vi "Dashboard Main.vi"() -> ()   [LabVIEW 2013]
uses:
  Common Code/Shooter State.ctl
  Common Code/Dashboard UDP/Camera Controls.ctl
  Common Code/Dashboard UDP/Gyro Controls.ctl
  Common Code/Dashboard UDP/PID Params.ctl
  Common Code/Dashboard UDP/Auton Controls.ctl
  Common Code/Dashboard UDP/Shooter Controls.ctl
  Common Code/Dashboard UDP/Encoder Controls.ctl
  Common Code/Dashboard UDP/Auto Shift Controls.ctl
  Common Code/Dashboard UDP/Roller Controls.ctl
  Common Code/Dashboard UDP/Shooter Indicators.ctl
  Common Code/Dashboard UDP/Auton Indicators.ctl
  Common Code/Dashboard UDP/Roller Indicators.ctl
  Common Code/IR Logic State.ctl
  Common Code/Dashboard UDP/Drive Indicators.ctl
  Common Code/Dashboard UDP/Halo Indicators.ctl
  Robot Code/Sensors/Encoder Data.ctl
  Robot Code/Sensors/Single Encoder Data.ctl
  Common Code/Vision Mode.ctl
  Common Code/Dashboard UDP/Fieldcentric Controls.ctl
  Common Code/Dashboard UDP/Roll Maneuver.ctl
  Robot Code/Drivetrain/DT Mode.ctl
  Common Code/Dashboard UDP Packet.ctl
  Common Code/Dashboard UDP/Omni Packet.ctl
  Common Code/Dashboard UDP/Indicator Packet.ctl
  <vilib>/event_ctls.llb/eventvkey.ctl
  Common Code/Change Detect Int.vi
  Common Code/Change Detect Double.vi
  Robot Code/Utilities/TimeManager.vi
  Common Code/Change Detect Boolean.vi
  <vilib>/Rock Robotics/WPI/Dashboard/WPI_DashboardLogging Global.vi
  <vilib>/Utility/config.llb/Write Key (String).vi
  <vilib>/Utility/config.llb/Write Key (I32).vi
  <vilib>/Utility/config.llb/NI_LVConfig.lvlib
panel:
  out "Maneuver Gyro Data":dbl[](array[numeric])
  in  "Shooter High":bool
  in  "PSI Good":bool
  in  "Shooter Ready":bool
  in  "Shooter State":T1
  in  "Color Components old":T2={"Hue"={70.0, 125.0}, "Sat"={39.0, 255.0}, "Val"={115.0, 255.0}} {"Val" scale=0.0..255.0; "Sat" scale=0.0..255.0; "Hue" scale=0.0..255.0 scale format="%#_3g"}
  out "Prefs Status":string
  out "High Priority User Data":string
  in  "Pressure/Blink Time":dbl=-1.0 caption="Blink (ms)"
  in  "Pressure/Deflicker":dbl=-1.0 caption="Deflicker (ms)"
  in  "Pressure/PID Setpoints D":dbl=-1.0 caption="D"
  in  "Pressure/PID Setpoints I":dbl=-1.0 caption="I"
  in  "Pressure/PID Setpoints P":dbl=-1.0 caption="P"
  in  "Pressure/PID Setpoints min":dbl=-1.0 caption="min"
  in  "Pressure/PID Setpoints max":dbl=-1.0 caption="max"
  in  "Pressure/Blink PSI Threshold":dbl=-1.0 caption="Blink Threshold"
  in  "Pressure/PSI Tolerance":dbl=-1.0 caption="Shoot\nThreshold"
  in  "Reload":bool
  in  "Save":bool
  out "Camera 2 IP":string="10.6.24.12"
  out "Camera IP":string="10.6.24.11"
  out "Heartbeat":dbl
  out "Connection LED":bool
  in  "stop":bool
  in  "Save Constants File":bool caption="Save"
  in  "Reload Constants File":bool caption="Reload"
  out "Image Message":string="Timeout in Camera Communications"
  in  "Rec Mode":enum32{"Stop", "Record", "Playback"}(radio)
  in  "Dashboard Tab":T3(tab)
  out "Shooter Retracted":bool caption="Retracted"
  out "Halo Mode":bool
  out "Roller Mode":bool
  out "Halo Indicators 2":T4
  out "Shooter State Indicator":bool
  out "Pressure/Shooter":dbl caption="Shooter"
  out "Shooter/High":bool caption="Pressure Setting"
  out "Pressure/Line":dbl(slide)=-1.0 caption="Tank" scale=50.0..120.0
  out "Pressure/Shooter":dbl(knob)=-1.0 caption="Shooter PSI" scale=30.0..60.0
  out "Shooter/State":T1
  out "Shooter/Trigger":bool caption="Trigger"
  out "Shooter/Release":bool caption="Release"
  out "Shooter/Add":bool caption="Add"
  out "Shooter/Ready":bool caption="Ready"
  out "Gyro Heading":dbl(knob) caption="Gyro" scale=0.0..359.0
  out "Roller Indicators 2":T5 caption="Rollers"
  out "Drive Indicators 2":T7 caption="Drive" {"Roller/Back Output" scale=-1.0..1.0; "Roller/Front Output" scale=-1.0..1.0; "Drive/Translation X" scale=-1.0..1.0; "Drive/Steer" scale=-1.0..1.0; "Drive/Throttle" scale=-1.0..1.0}
  out "Gyro Heading":dbl(knob) caption="Gyro" scale=0.0..359.0
  in  "Disable Compressor":bool caption="Disable\nCompressor"
  in  "IR Halo Sustain Time":dbl caption="IR Halo Sustain"
  out "Halo Indicators":T8
  in  "Encoder":T9={"Encoders/Reset"=FALSE, "Encoders/Omni Constant"=0.000546, "Encoders/Omni Tick Constant"=10.27628431, "Encoders/Left Constant"=0.000546, "Encoders/Right Constant"=0.000546, "Encoders/Right Tick Constant"=1.0}
  out "Drive/Gear":dbl caption="Gear"
  in  "Pressure/Compressor Delay":dbl=500.0 caption="Delay"
  in  "Pressure/Compressor Min Voltage":dbl=7.0 caption="Min Volts"
  in  "Drive/Ramp X":dbl=250.0 caption="Ramp X (ms)"
  in  "Drive/Ramp Y":dbl=250.0 caption="Ramp Y (ms)"
  out "IR Dist/Line Detected Right":bool caption="Right Line"
  out "IR Dist/Line Detected Left":bool caption="Left Line"
  in  "Drive/Battery Cutoff":dbl=6.0 caption="Drive Min Volts"
  in  "Shooter":T10={"Shooter/Reset Time"=500.0, "Shooter/Release Delay"=150.0, "Shooter/Pressure Steady Time"=0.0, "Shooter/Misfire Delay"=2000.0, "Shooter/Ball Settle Time"=500.0, "Shooter/Line IR Delay"=300.0, "Pressure/Upper PSI Time"=500.0, "Pressure/Lower PSI Time"=500.0, "Shooter/Punch Delay"=-150.0, "Shooter/Target Pressure"=43.0, "Pressure/Line B"=-57.077, "Pressure/Line M"=33.41, "Pressure/Shooter M"=33.41, "Pressure/Shooter B"=-57.077, "Halo Time"=150.0, "Soft Release Delay"=0.0, "Soft Unpin Delay"=0.0, "Soft Shoot Delay"=0.0, "Toss Release Time"=0.0} caption="Soft Shoot"
  in  "Auto Shift":T11={"AutoShift/Upshift Throttle Accel"=-2.0, "AutoShift/Speed Threshold"=5.0, "AutoShift/Upshift Throttle"=0.8, "AutoShift/Upshift Accel"=0.5, "AutoShift/Downshift Accel"=-1.2, "AutoShift/Downshift Throttle"=0.15, "AutoShift/Delay"=1000.0, "AutoShift/Enabled"=TRUE}
  in  "Rollers":T12={"Roller/Load IRs Verify Time"=150.0, "Roller/Center IR Latch Time"=500.0, "Roller/Speed Front"=0.8, "Roller/Speed Back"=0.3, "Roller/Entry Timeout"=750.0, "Roller/To Center Timeout"=2000.0, "Roller/Sustain Time"=5000.0, "Roller/Verify Center Time"=750.0}
  out "Shooter Indicators":T13={"Pressure/Line"=-1.0, "Pressure/Shooter"=-1.0, "Shooter/Release"=FALSE, "Shooter/Trigger"=FALSE, "Shooter/Retracted"=FALSE, "Shooter/Ready"=FALSE, "Shooter/Add"=FALSE, "Shooter/State"=enum."Wait", "Shooter/Punch"=FALSE, "Shooter/High"=FALSE, "Shooter/AutoPunch"=FALSE}
  out "Roller Indicators":T5
  out "Drive Indicators":T7 {"Roller/Back Output" scale=-1.0..1.0; "Roller/Front Output" scale=-1.0..1.0; "Drive/Translation X" scale=-1.0..1.0; "Drive/Steer" scale=-1.0..1.0; "Drive/Throttle" scale=-1.0..1.0}
  out "Encoder Data":T14 {"Omni"."Ticks" format="%#.6g"; "Right"."Ticks" format="%#.6g"; "Left"."Ticks" format="%#.6g"}
  in  "Low PSI":dbl=52.0
  in  "Center Omni Drive Delay":dbl
  in  "Controller/Strafe Correction":bool=TRUE caption="Strafe Correct"
  in  "Auton":T16={"Auton/Left Shoot X-Coord"=-4.0, "Auton/Right Shoot X-Coord"=4.0, "DistDrive/Distance Stop Threshold"=0.25, "DistDrive/Max Stop Speed"=0.5, "Auton/Back Piston Time"=500.0, "Auton/Manual Hot"=FALSE, "Auton/Manual Hot Right"=FALSE, "Default X PID"={"max"=1.0, "min"=-1.0, "P"=0.36, "I"=0.0, "D"=0.0}, "Default Y PID"={"max"=1.0, "min"=-1.0, "P"=0.7, "I"=0.0, "D"=0.001}, "Half Over Delay"=0.0}
  out "Auton/Files":string
  out "Auton Indicators":T18
  out "Vision Mode":T19 caption="Vision Mode (Reported by Robot)"
  in  "Normal Vision":bool=TRUE
  in  "Extreme Left":bool
  in  "Extreme Right":bool
  out "Vision Mode Cam":T19 caption="Reported Vision Mode"
  in  "Camera":T20={"Camera/View Angle X"=66.5, "Camera/Goal Track Timeout"=120.0, "Camera/View Angle Y"=49.0, "Camera/Goal Exposure"=0.0, "Camera/Vision Receive Timeout"=120.0, "Camera/Offset 1"=-35.0, "Camera/Offset 2"=35.0}
  in  "Cam 2 Enable":bool=TRUE
  out "Auton/Right Hot":bool
  out "Auton/Left Hot":bool
  out "Cam2 FPS":dbl format="%#.1g"
  out "Cam2 Mbps":dbl format="%#.1g"
  out "Cam2 LED":bool
  in  "Camera Settings":T21={"Frame Rate"=30, "Compression"=30, "Size"=1} {"Frame Rate" scale=1.0..30.0; "Size" items=["640x480", "320x240", "160x120"]}
  out "Camera Image":T22(plugin-control)
  in  "Cam 1 Enable":bool=TRUE
  out "Camera Image 2":T22(plugin-control)
  out "Mbps 2":bool
  out "Cam1 Mbps":dbl format="%#.1g"
  out "Cam1 FPS":dbl format="%#.1g"
  in  "DB Camera Config":bool
  in  "Test Slider":dbl(slide) scale=0.0..100.0 scale format="%#_3g"
  in  "On/Off":bool caption="Solenoid"
  in  "Test Name":u16(ring) items=["Select the test to run...", "Example Test", "-------------------------------", "List of tests is built in robot code.", "Replace with your own automated tests."]
  in  "Test Tree":string(tree)
  in  "Motor":cluster{"Value":dbl, "Enable":bool} {"Value" scale=-1.0..1.0 scale format="%#_3g"}
  out "Progress":T23 {"Test Progress" scale=0.0..100.0}
  in  "Rev/Fwd":cluster{"Forward":bool, "Reverse":bool}
  in  "Test Ring":u16(ring) items=["Auto", "Fixed indoor", "Fixed outdoor 1", "Fixed outdoor 2", "Fixed fluorescent 1", "Fixed fluorescent 2", "Hold current"]
  out "Tree":string(tree)
  in  "Listbox":i32(listbox)
  out "Warnings List":string
  out "Preferences Count":i32
  in  "Gyro":T24={"Gyro/Angle Tolerance"=2.0, "Gyro/Steer Closeness Threshold"=10.0, "Steer PID"={"max"=0.8, "min"=-0.8, "P"=0.04, "I"=0.0, "D"=0.0}, "Steer Close PID"={"max"=0.7, "min"=-0.7, "P"=0.04, "I"=0.0, "D"=0.002}}
  out "Gyro/In Range":bool
  out "Gyro/Steer Target":dbl
  out "Gyro Heading":dbl(knob) scale=0.0..359.0
  out "Vision Mode Goal Tab":T19 caption="Vision Mode"
  in  "Cam 1/2":bool
  out "Goal Mask":T22(plugin-control)
  out "Goal Camera Image":T22(plugin-control)
  in  "Score Cutoff":dbl(slide)=54.248366013071895 scale=0.0..100.0
  in  "HSV Filter":T25={"Hue min"=100.0, "Hue max"=125.0, "Sat min"=60.0, "Sat max"=255.0, "Lum min"=155.0, "Lum max"=255.0}
  in  "Stick Deadband":dbl
  out "Angle Graph":T26(graph)
  out "Drive Graph":cluster{i32, "Timestep(ms)":i32, dbl[][]}(graph)
  in  "Roll":T27
  in  "Fieldcentric":T28
  in  "Radius Throttle":bool
  out "Drivetrain Mode":T29
  out "Time/100ms loop exec time":dbl
  in  "Finish":bool caption="Self Destruct"
  in  "Abort":bool caption="Self Destruct"
  out "Mode":T30(ring)=enum."Auto Disabled"
  # "Pressure PID"
  # "psi"
  # "psi"
  # "Shooter"
  # "IR"
  # "Encoders"
  # "Auto Shift"
  # "Compressor"
  # "Feet"
  # "Line"
  # "Shooter"
  # "Down"
  # "Up"
  # "IR"
  # "Left"
  # "Front"
  # "Right"
  # "Battery"
  # "2"
  # "1"
  # "Goal Tracking"
  # "DRIVER [USB 1]"
  # "Manipulator [USB 2]"
  # "DRIVER [USB 1]"
  # "Manipulator [USB 2]"
  # "JOYSTICK"
  # "CONTROLS"
  # "GAMEPAD"
  # "CONTROLS"
  # "GAMEPAD"
  # "CONTROLS"
  # "GAMEPAD"
  # "CONTROLS"
  # "Joystick"
  # "A 1-X    \tThrottle\t\nA 2-Y     Lateral Throttle (Omni)\nA 3-Z     Spin\nA +/-     Omni Traction Switch\n\n1\t            Gear Shift (INA)\n2\t            Shoot (RAS)\n3\t            Collect Ball (Front)\t(INA)\n4\t            Collect Ball (Rear) (INA)\n5\t            Trigger\n6\t            Reset Gyro\n7\t            Front Arm Up/Down \n8\t            Back Arm Up/Down\n9\t            F Roller In\n10\t\t         R Roller In\n11           F Roller Out\n12           R Roller Out\n\t\t\nUP\t           Add Pressure\t\nDOWN\t    Release Pressure\t\nLEFT\t        Goal Offset LEFT\nRIGHT\t\t    Goal Offset RIGHT"
  # "11           \t\n12\t\t\n\n\n\n1\t\t\n2\t            \n3\t            Warmup\t\n4\t\t\n5             \n6\t            \t\n7\t            \n8\t\n9\t            Camera Search\t*\n10\t          Auto Ball\t*\n11\t          \t\n12\t\n\t\nUP\t\t\nDOWN\t\t\nLEFT\t\t\nRIGHT"
  # "Joystick"
  # "11    \t      Throttle\t\n12\t          Steer\n\n1\t            Roll maneuver left\n2\t            Shoot\t& (AS)\n3\t            \tRoll maneuver right\n4\t            Goal Steer\t& (AS)\n5\t            Manual low gear / Gear          \n               shift\n6\t            Omni Toggle\t\n7\t            Strafe Left \n8\t            Strafe Right\n9\t             \n10\t\t\n11          \t\n12\n\t\n\n\t\nUP\t          \t\nDOWN\t    \t\nLEFT\t        \t\nRIGHT"
  # "11        Y-High/Low PSI Set\n12\t  R= Hold Ball L=Carry Two               \n1\t\t        SHIFT Alt Ctrl [...]\n2\t         Shoot\t\n3\t         Ready Shooter\t\n4\t\t        Invert Halo\n5          Front Roller-Fwds\n                [manual Trigger*]\n6\t    \t\n7\t         Front Roller-Backwds\t\n                [Line Shoot]\n8\t     \n9\t        Auto Halo* \n         [Manual Halo Setting] \n10\t       Auto Roller\t*\n11\t      \t\n12\t       Recal Gyro (only when    disabled)\n\nUP\t\t       Load Front [+ Air]\nDOWN\t Reset Load [- Air]\nLEFT\t\t    Load Front [Reset Air]\nRIGHT   Toss Ball"
  # "Buttons"
  # "Buttons"
  # "D-Pad"
  # "D-Pad"
  # "(INA) If Not Automated"
  # "* Toggle"
  # "AUTON SELECT: With robot disabled, press button 9 + button 2 to go down file list\n                                                                         button 9 + button 4 to go up file list"
  # "(RAS) Runs Automatic Sequence"
  # "* Toggle"
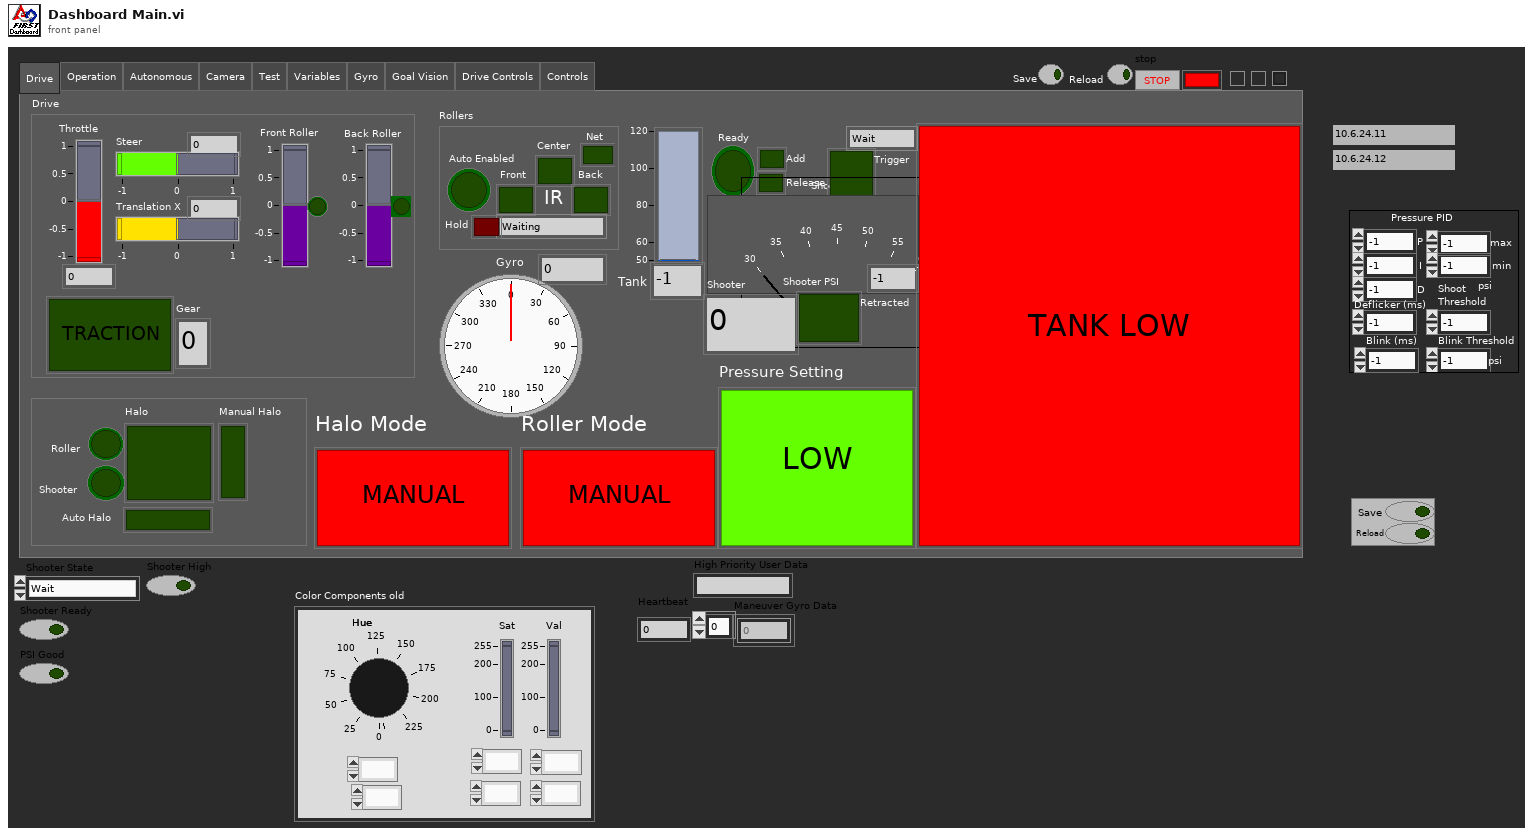
[diagram p1: front panel]
types:
  T1 = typedef "Shooter State.ctl" = enum16{"Wait", "Fill Piston", "Lift Halo", "Trigger", "Reset", "Soft Release", "Soft Unpin", "Soft Refill", "Soft Shoot", "Toss Prep", "Toss Release"}
  T2 = cluster{"Hue":cluster{dbl, dbl}, "Sat":cluster{dbl, dbl}, "Val":cluster{dbl, dbl}}
  T3 = enum32{"Drive", "Operation", "Autonomous", "Camera", "Test", "Variables", "Gyro", "Goal Vision", "Drive Controls", "Controls"}
  T4 = cluster{"Halo":bool, "Roller Halo":bool, "Shooter Halo":bool, "Auto Halo":bool, "Manual Halo":bool}
  T5 = typedef "Roller Indicators.ctl" = cluster{"Roller/Front IR":bool, "Roller/Center IR":bool, "Roller/Back IR":bool, "Roller/IR State":T6, "Roller/Auto Enabled":bool, "Roller/Hold":bool, "Roller/Net Solenoid":bool}
  T6 = typedef "IR Logic State.ctl" = enum16{"Waiting", "Requested", "Loading", "Full", "Wait for Center", "Carry", "Full Carry", "Holding"}
  T7 = typedef "Drive Indicators.ctl" = cluster{"Drive/Throttle":dbl, "Drive/Steer":dbl, "Drive/Translation X":dbl, "Drive/Omni":bool, "Roller/Front Output":dbl, "Roller/Back Output":dbl, "Roller/Front Solenoid":bool, "Roller/Back Solenoid":bool, "Drive/Gear":dbl}
  T8 = typedef "Halo Indicators.ctl" = cluster{"Halo":bool, "Roller Halo":bool, "Shooter Halo":bool, "Auto Halo":bool, "Manual Halo":bool}
  T9 = typedef "Encoder Controls.ctl" = cluster{"Encoders/Reset":bool, "Encoders/Omni Constant":dbl, "Encoders/Omni Tick Constant":dbl, "Encoders/Left Constant":dbl, "Encoders/Right Constant":dbl, "Encoders/Right Tick Constant":dbl}
  T10 = typedef "Shooter Controls.ctl" = cluster{"Shooter/Reset Time":dbl, "Shooter/Release Delay":dbl, "Shooter/Pressure Steady Time":dbl, "Shooter/Misfire Delay":dbl, "Shooter/Ball Settle Time":dbl, "Shooter/Line IR Delay":dbl, "Pressure/Upper PSI Time":dbl, "Pressure/Lower PSI Time":dbl, "Shooter/Punch Delay":dbl, "Shooter/Target Pressure":dbl, "Pressure/Line B":dbl, "Pressure/Line M":dbl, "Pressure/Shooter M":dbl, "Pressure/Shooter B":dbl, "Halo Time":dbl, "Soft Release Delay":dbl, "Soft Unpin Delay":dbl, "Soft Shoot Delay":dbl, "Toss Release Time":dbl}
  T11 = typedef "Auto Shift Controls.ctl" = cluster{"AutoShift/Upshift Throttle Accel":dbl, "AutoShift/Speed Threshold":dbl, "AutoShift/Upshift Throttle":dbl, "AutoShift/Upshift Accel":dbl, "AutoShift/Downshift Accel":dbl, "AutoShift/Downshift Throttle":dbl, "AutoShift/Delay":dbl, "AutoShift/Enabled":bool}
  T12 = typedef "Roller Controls.ctl" = cluster{"Roller/Load IRs Verify Time":dbl, "Roller/Center IR Latch Time":dbl, "Roller/Speed Front":dbl, "Roller/Speed Back":dbl, "Roller/Entry Timeout":dbl, "Roller/To Center Timeout":dbl, "Roller/Sustain Time":dbl, "Roller/Verify Center Time":dbl}
  T13 = typedef "Shooter Indicators.ctl" = cluster{"Pressure/Line":dbl, "Pressure/Shooter":dbl, "Shooter/Release":bool, "Shooter/Trigger":bool, "Shooter/Retracted":bool, "Shooter/Ready":bool, "Shooter/Add":bool, "Shooter/State":T1, "Shooter/Punch":bool, "Shooter/High":bool, "Shooter/AutoPunch":bool}
  T14 = typedef "Encoder Data.ctl" = cluster{"Avg Distance L/R":dbl, "Avg Speed L/R":dbl, "Left":T15, "Right":T15, "Omni":T15}
  T15 = typedef "Single Encoder Data.ctl" = cluster{"Distance":dbl, "Speed":dbl, "Ticks":dbl}
  T16 = typedef "Auton Controls.ctl" = cluster{"Auton/Left Shoot X-Coord":dbl, "Auton/Right Shoot X-Coord":dbl, "DistDrive/Distance Stop Threshold":dbl, "DistDrive/Max Stop Speed":dbl, "Auton/Back Piston Time":dbl, "Auton/Manual Hot":bool, "Auton/Manual Hot Right":bool, "Default X PID":T17, "Default Y PID":T17, "Half Over Delay":dbl}
  T17 = typedef "PID Params.ctl" = cluster{"max":dbl, "min":dbl, "P":dbl, "I":dbl, "D":dbl}
  T18 = typedef "Auton Indicators.ctl" = cluster{"DistDrive/Steer":bool, "DistDrive/Y Check":bool, "Auton/Left Hot":bool, "Auton/Right Hot":bool, "DistDrive/Y Dist":dbl, "DistDrive/Y Target":dbl, "DistDrive/X Dist":dbl, "DistDrive/X Target":dbl, "Gyro Heading":dbl, "DistDrive/Steer Target":dbl, "DistDrive/X Check":bool, "Auton/Hot Found":bool, "Auton/Goals Used":dbl, "Auton/Total Commands":dbl, "Auton/Current Command":dbl, "Auton/File":dbl}
  T19 = typedef "Vision Mode.ctl" = enum16{"Normal", "Extreme Left", "Extreme Right"}
  T20 = typedef "Camera Controls.ctl" = cluster{"Camera/View Angle X":dbl, "Camera/Goal Track Timeout":dbl, "Camera/View Angle Y":dbl, "Camera/Goal Exposure":dbl, "Camera/Vision Receive Timeout":dbl, "Camera/Offset 1":dbl, "Camera/Offset 2":dbl}
  T21 = cluster{"Frame Rate":i32, "Compression":i32, "Size":u16}
  T22 = typedef "IMAQ Image.ctl" = refnum<image>
  T23 = cluster{"Test Progress":u8, "Test Progress Text":string}
  T24 = typedef "Gyro Controls.ctl" = cluster{"Gyro/Angle Tolerance":dbl, "Gyro/Steer Closeness Threshold":dbl, "Steer PID":T17, "Steer Close PID":T17}
  T25 = cluster{"Hue min":dbl, "Hue max":dbl, "Sat min":dbl, "Sat max":dbl, "Lum min":dbl, "Lum max":dbl}
  T26 = cluster{i32, "Timestep(ms)":i32, "Maneuver Gyro Data":dbl[]}[]
  T27 = typedef "Roll Maneuver.ctl" = cluster{"X 1":dbl, "Y 1":dbl, "Y 2":dbl, "X 2":dbl, "Y 3":dbl, "X 3":dbl, "Time 1":i32, "Time 2":i32, "Time 3":i32, "Angle Start":dbl, "Angle End":dbl, "Angle Linearity":dbl}
  T28 = typedef "Fieldcentric Controls.ctl" = cluster{"Relative Angle":bool, "Point Robot":bool, "X/Y ratio low":dbl, "Steering Gain":dbl, "Force Omni Down":bool, "Enable":bool, "X/Y ratio high":dbl}
  T29 = typedef "DT Mode.ctl" = enum16{"Manual", "Gyro Steer", "Distance Drive", "Fieldcentric", "Roll Maneuver", "Alt Roll Maneuver"}
  T30 = enum8{"Tele-Op Disabled", "Tele-Op Enabled", "Auto Disabled", "Auto Enabled", "Test Disabled", "Test Enabled", ""}
  T31 = typedef "Image Type" = u32
  T32 = typedef "NI_LVConfig.lvlib/Config Data RefNum.ctl" = refnum<k1>
  T33 = typedef "Goal Info.ctl" = cluster{"Found?":bool, "Target Center":cluster{"X":dbl, "Y":dbl}, "Distance (ft)":dbl, "Hot?":bool, "Left?":bool, "Camera":i16}
  T34 = cluster{"Vision Target":T33, "Vision Target":T33, "Vision Target":T33}
  T35 = cluster{"Competition mode":bool, "Robot Link":bool, "Autonomous":bool, "Enabled":bool, "E-Stop":bool, "Simulated":bool, "TestMode":bool, "Docked Window":bool}
  T36 = typedef "eventvkey.ctl" = enum16{"ASCII", "Enter", "Return", "Shift", "Ctrl", "Alt", "Cmd", "Opt", "Caps", "NumLock", "Clear", "Break", "Up", "Down", "Left", "Right", "Insert", "Delete", "Home", "End", "PageUp", "PageDown", "Escape", "Help", "Pause", "ScrollLock", "F1", "F2", "F3", "F4", "F5", "F6", "F7", "F8", "F9", "F10", "F11", "F12", "F13", "F14", "F15", "F16", "F17", "F18", "F19", "F20", "F21", "F22", "F23", "F24", "Play", "VolumeUp", "VolumeDown", "Mute", "Two Byte Char"}
  T37 = cluster{"Image Size":bool, "Image Type":bool, "Pixel Value":bool, "ROI Information":bool, "Zoom Factor":bool}
  T38 = typedef "Omni Packet.ctl" = cluster{"Type":i32, "data string":string}
  T39 = typedef "Dashboard UDP Packet.ctl" = cluster{"Camera":T20, "Gyro":T24, "Encoder":T9, "Auto Shift":T11, "Auton":T16, "Drive/Ramp X":dbl, "Drive/Ramp Y":dbl, "Drive/Battery Cutoff":dbl, "Pressure/Compressor Min Voltage":dbl, "Pressure/Compressor Delay":dbl, "Controller/Strafe Correction":bool, "Shooter":T10, "Rollers":T12, "Abort":bool, "Finish":bool, "IR Halo Sustain Time":dbl, "Disable Compressor":bool, "Center Omni Drive Delay":i32, "Vision Mode":T19, "Radius Throttle":bool, "Fieldcentric":T28, "Roll":T27, "Stick Deadband":dbl}
  T40 = typedef "Indicator Packet.ctl" = cluster{"Gyro/Steer Target":dbl, "Gyro/In Range":bool, "Gyro Heading":dbl, "Auton/Files":string, "Auton Indicators":T18, "Heartbeat":dbl, "100ms Loop Time":i32, "IR Dist/Line Detected Left":bool, "IR Dist/Line Detected Right":bool, "Roller Indicators":T5, "Shooter/Indicators":T13, "Halo/Indicators":T8, "Drive Indicators":T7, "Encoder Data":T14, "Vision Mode ":T19, "Drivetrain Mode":T29}
  T41 = typedef "Named Control.ctl" = cluster{"Name":string, "Control":refnum<vi>, "Type":enum16{"Boolean", "Double"}}[]
  T42 = cluster{i32, "Timestep(ms)":i32, "Angle Array":dbl[]}
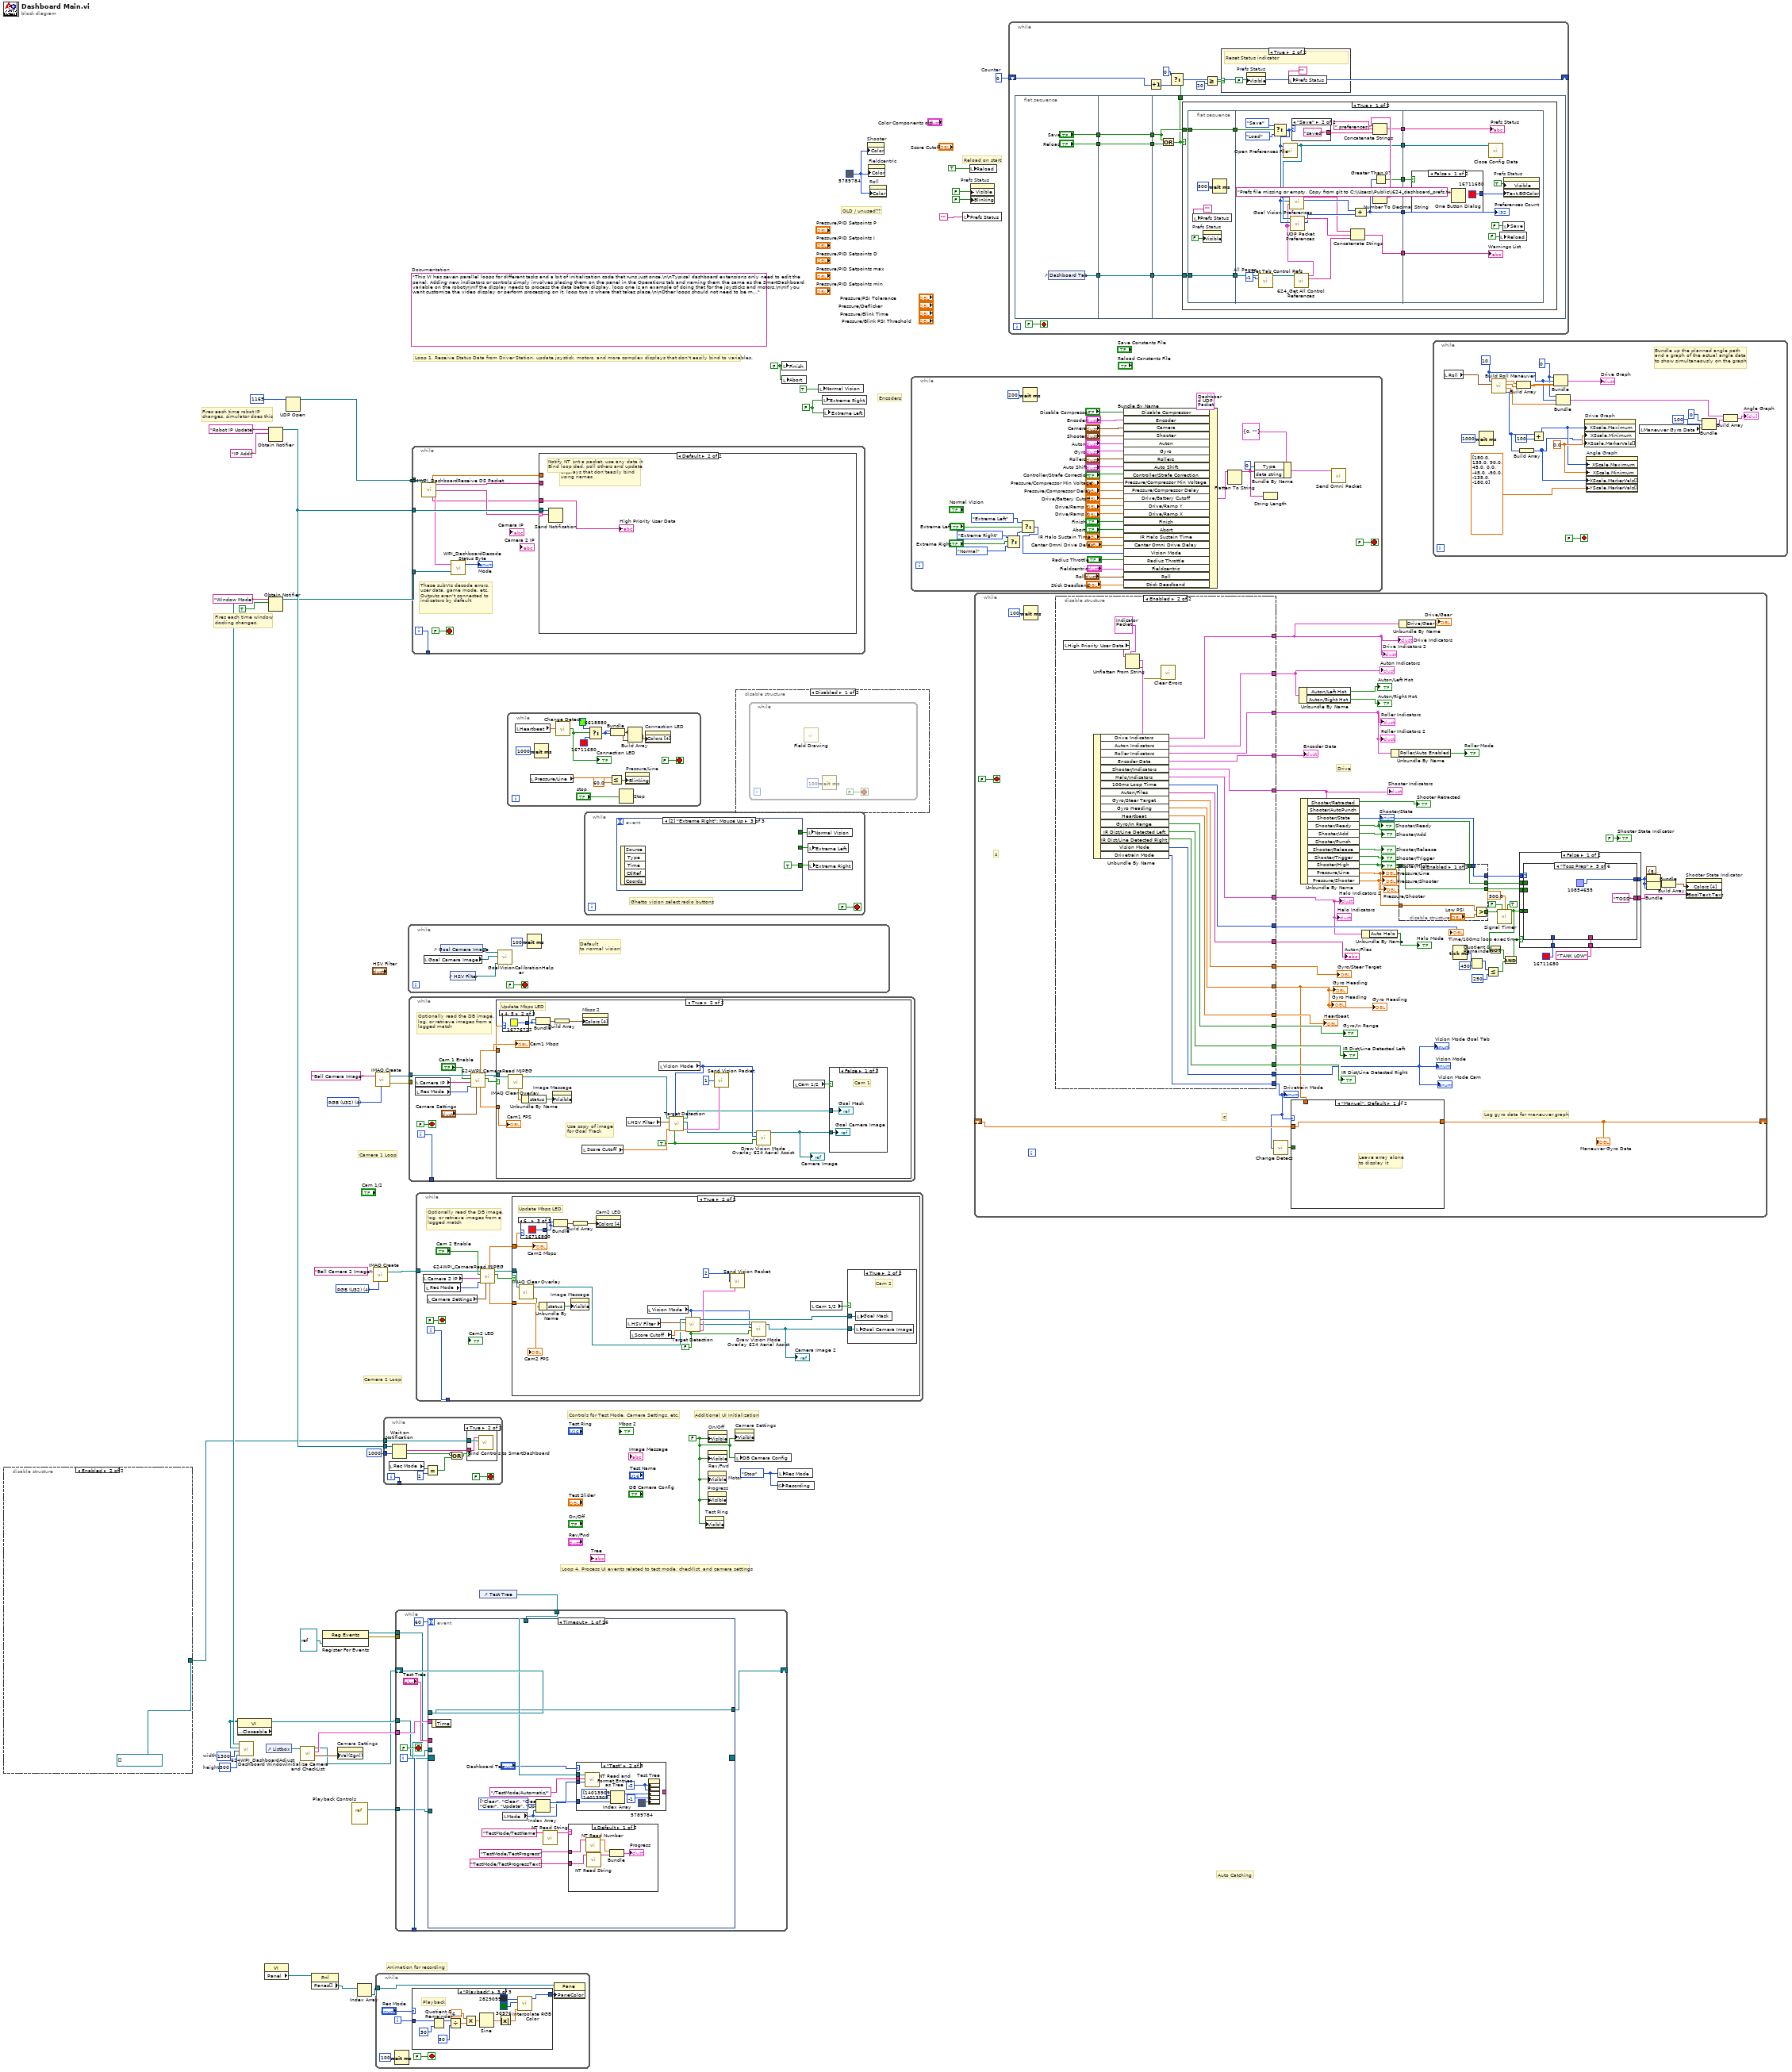
[diagram p0: block diagram]
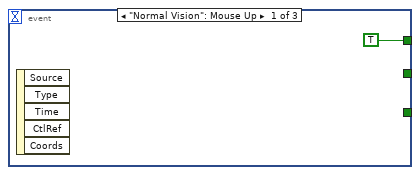
[diagram p2: hidden frame]
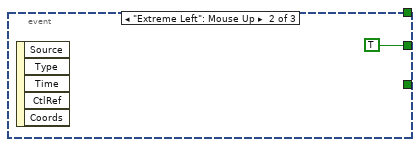
[diagram p3: hidden frame]
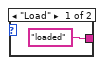
[diagram p5: hidden frame]
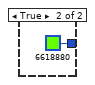
[diagram p6: hidden frame]
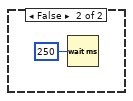
[diagram p7: hidden frame]
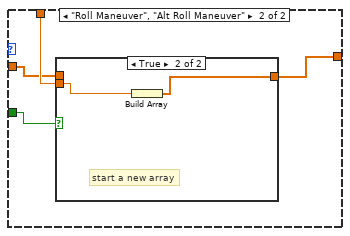
[diagram p9: hidden frame]
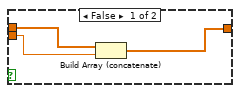
[diagram p10: hidden frame]
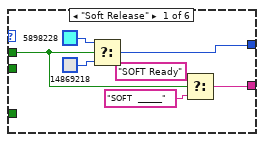
[diagram p11: hidden frame]
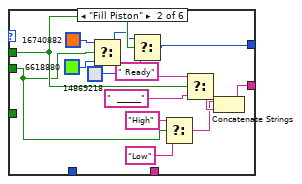
[diagram p12: hidden frame]
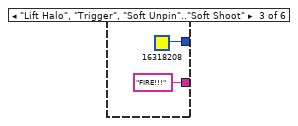
[diagram p13: hidden frame]
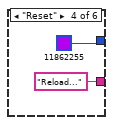
[diagram p14: hidden frame]
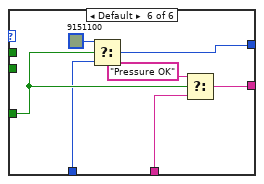
[diagram p15: hidden frame]
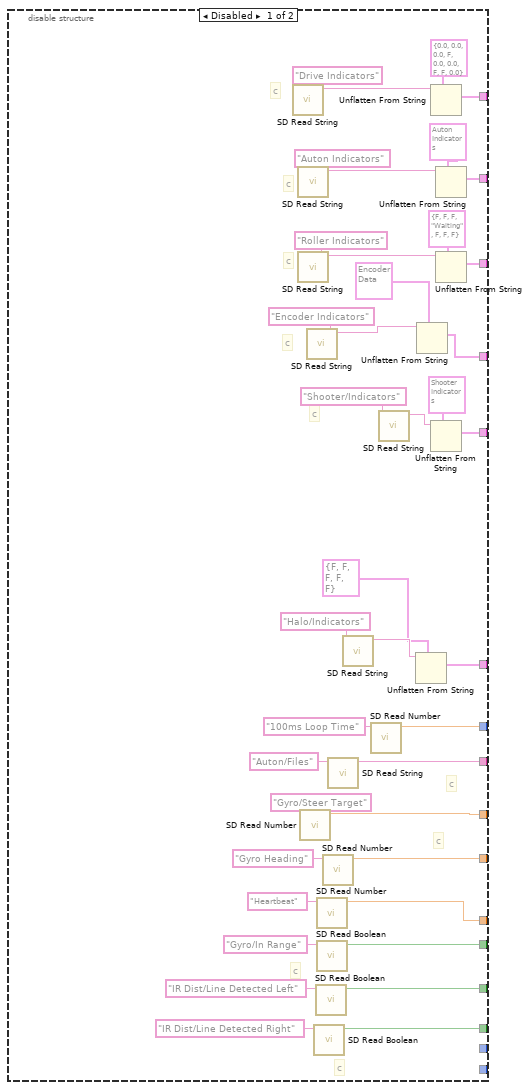
[diagram p17: hidden frame]
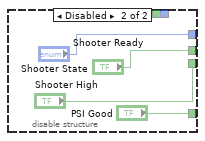
[diagram p18: hidden frame]
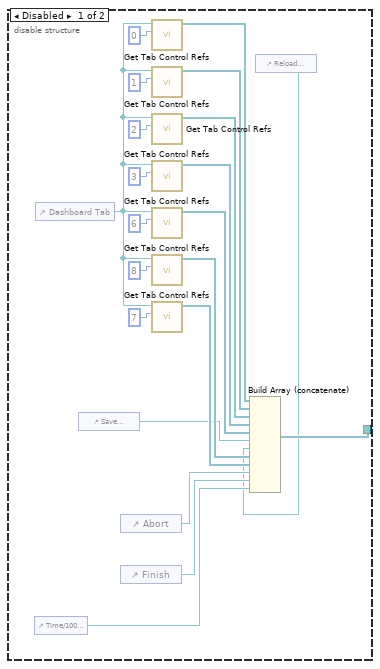
[diagram p19: hidden frame]
diagram:
  w1 = u32 5789784
  w3 = FALSE ("Finish")
  w4 = 0  # Counter
  w10 = FALSE ("Finish")
  w18 = T31 4 items=["Grayscale (U8)", "Grayscale (I16)", "Grayscale (SGL)", "Complex (CSG)", "RGB (U32)", "HSL (U32)", "RGB (U64)"] ("Image Type")
  w22 = enum32{"Stop", "Record", "Playback"}."Stop" ("Rec Mode")
  w24 = 500  # height
  w25 = 1300  # width
  w33 = FALSE ("Visible")
  (unwired) "This VI has seven parallel loops for different tasks and a bit of initialization code that runs just once.\n\nTypical dashboard extensions only need to edit the panel. Adding new indicators or controls simply involves placing them on the panel in the Operations tab and naming them the same as the SmartDashboard variable on the robot\n\nIf the display needs to process the data before display, loop one is an example of doing that for the joysticks and motors.\n\nIf you want customize the video display or perform processing on it, loop two is where that takes place.\n\nOther loops should not need to be modified. They are pretty standard, and document the task they perform."  # Documentation
  w41 = T31 4 items=["Grayscale (U8)", "Grayscale (I16)", "Grayscale (SGL)", "Complex (CSG)", "RGB (U32)", "HSL (U32)", "RGB (U64)"] ("Image Type")
  # "Reload on start"
  # "OLD / unused??"
  # "Encoders"
  # "Auto Catching"
  # "Camera 2 Loop"
  # "Camera 1 Loop"
  # "Controls for Test Mode, Camera Settings, etc."
  # "Additional UI Initialization"
  # "Animation for recording"
  # "Fires each time robot IP\nchanges, simulator does this"
  # "Fires each time window\ndocking changes."
  # "Loop 4. Process UI events related to test mode, checklist, and camera settings"
  # "Loop 1. Receive Status Data from Driver Station, update joystick, motors, and more complex displays that don't easily bind to variables."
  n1 = disable-structure shown="Enabled" {
    disable-tunnel: [w57 refnum<vi>[] []] -> w11
    frame Disabled {
      n2 = control-ref of="Time/100ms loop exec time"() -> (w45:refnum<vi>)
      n3 = control-ref of="Dashboard Tab"() -> (w46:refnum<vi>)
      n4 = control-ref of="Save Constants File"() -> (w49:refnum<vi>)
      n5 = control-ref of="Abort"() -> (w48:refnum<vi>)
      n6 = control-ref of="Finish"() -> (w47:refnum<vi>)
      n7 = call <vilib>:"Get Tab Control Refs.vi"("Page Index"=0, "TabControl in"=w46) -> ("ControlsOnPage"=w52:refnum<vi>[])  [unwired: 9 in]
      n8 = call <vilib>:"Get Tab Control Refs.vi"("Page Index"=1, "TabControl in"=w46) -> ("ControlsOnPage"=w51:refnum<vi>[])  [unwired: 9 in]
      n9 = call <vilib>:"Get Tab Control Refs.vi"("Page Index"=2, "TabControl in"=w46) -> ("ControlsOnPage"=w56:refnum<vi>[])  [unwired: 9 in]
      n10 = call <vilib>:"Get Tab Control Refs.vi"("Page Index"=3, "TabControl in"=w46) -> ("ControlsOnPage"=w54:refnum<vi>[])  [unwired: 9 in]
      n11 = call <vilib>:"Get Tab Control Refs.vi"("Page Index"=6, "TabControl in"=w46) -> ("ControlsOnPage"=w53:refnum<vi>[])  [unwired: 9 in]
      n12 = call <vilib>:"Get Tab Control Refs.vi"("Page Index"=8, "TabControl in"=w46) -> ("ControlsOnPage"=w55:refnum<vi>[])  [unwired: 9 in]
      n13 = call <vilib>:"Get Tab Control Refs.vi"("Page Index"=7, "TabControl in"=w46) -> ("ControlsOnPage"=w50:refnum<vi>[])  [unwired: 9 in]
      n14 = control-ref of="Reload Constants File"() -> (w44:refnum<vi>)
      n15 = Build Array (concatenate)(w52, w51, w56, w54, w53, w49, w44, w55, w50, w48, w47, w45) -> (w57:refnum<vi>[])
    }
    frame Enabled {
    }
  }
  n16 = property class="VI" props=["Front Panel.Closeable"]() -> (reference out=w21:refnum<vi>)  [unwired: 2 in, 2 out]
  n17 = property class="VI"() -> ("Panel"=w30:refnum<vi>)  [unwired: 2 in, 2 out]
  n18 = control-ref of="Listbox"() -> (w12:refnum<vi>)
  n19 = Obtain Notifier(name (unnamed)="Robot IP Update", notification data type="IP Addr" ("name (unnamed)")) -> (notifier out=w36:refnum<notifier>)  [unwired: 2 in, 2 out]
  n20 = Obtain Notifier(name (unnamed)="Window Mode", notification data type=TRUE) -> (notifier out=w23:refnum<notifier>)  [unwired: 2 in, 2 out]
  n21 = call "624WPI_DashboardAdjust Dashboard Window.vi"("height"=w24, "width"=w25, "reference in"=w21, "Notifier in"=w23) -> ()  [unwired: 8 in]
  n22 = UDP Open(11:u16 1165 ("port")) -> (port=w42:refnum<k16>)  [unwired: 2 in, 4 out]
  n23 = call "Initialize Camera and CheckList.vi"("ListBox in"=w12) -> ("Cluster"=w15:cluster{"value":i32, "value":i32, "index":i32}, "Array"=w14:cluster{string[]}[], "File Refnum"=w13:T32)  [unwired: 8 in]
  n24 = property class="Pnl"(reference=w30) -> ("Panes[]"=w31:refnum<vi>[])  [unwired: 1 in, 2 out]
  n25 = register-events(refnum<vi> refnum) -> (reference out=w28:refnum<event-registration>, error out=w27:errorcluster)  [unwired: 2 in]
  n26 = property on="Camera Settings" class="Clust (strict)"("Val(Sgnl)"=w15) -> ()  [unwired: 2 in, 2 out]
  n27 = vi-ref "Playback Controls.vi"() -> (w16:refnum<vi>)
  n28 = Index Array(array=w31) -> (element=w29:refnum<vi>)  [unwired: 1 in]
  n29 = call "IMAQ Create"("Image Name"="Ball Camera 2 Image", "Image Type"=w18) -> ("New Image"=w19:T22)  [unwired: 2 in, 2 out]
  n30 = call "IMAQ Create"("Image Name"="Ball Camera Image", "Image Type"=w41) -> ("New Image"=w40:T22, "error out"=w39:errorcluster)  [unwired: 2 in, 1 out]
  n31 = while {
    tunnel: w29 -> [w67]
    i -> [w70]
    stop <- FALSE stop-if-true
    n32 = Wait (ms)(milliseconds to wait=u32 100) -> ()  [unwired: 1 out]
    n33 = case shown="\"Playback\"" "Rec Mode" {
      tunnel: w70 -> [_ _ w85]
      tunnel: [u32 2829099 ("Base Color") u32 11141120 ("Target Color") w77] -> w66
      frame "Stop", Default {
        # "Reset the color, extra updates don't cost much"
      }
      frame "Record" {
      }
      frame "Playback" {
        # "Playback"
        n34 = Quotient & Remainder(x=w85, y=u32 50 ("milliseconds to wait")) -> (x-y*floor(x/y)=w81:u32)  [unwired: 1 out]
        n35 = Divide(x=w81, y=u32 50 ("milliseconds to wait")) -> (x/y=w78:dbl)
        n36 = Multiply(x=6.283185307179586, y=w78) -> (x*y=w83:dbl)
        n37 = Sine(x=w83) -> (sin(x)=w82:dbl)
        n38 = Absolute Value(x=w82) -> (abs(x)=w76:dbl)
        n39 = call "Interpolate RGB Color.vi"("Proportion"=w76, "Target Color"=u32 30976, "Base Color"=u32 2829099) -> ("Result Color"=w77:u32)  [unwired: 8 in]
      }
    }
    n40 = property class="Pane"(reference=w67, "PaneColor"=w66) -> ()  [unwired: 1 in, 2 out]
  }
  n41 = while {
    tunnel: w11 -> [w96]
    tunnel: w36 -> [w94]
    tunnel: [w92] -> _
    tunnel: u32 1000 ("milliseconds to wait") -> [w91]
    i -> [w92]
    stop <- FALSE stop-if-true
    n42 = local read "Rec Mode"() -> (w87:enum32{"Stop", "Record", "Playback"})
    n43 = Wait on Notification(notifier=w94, timeout in ms (-1)=w91) -> (notification=w93:string, timed out?=w89:bool)  [unwired: 2 in, 2 out]
    n44 = Equal?(x=w87, y=u16 2 ("Rec Mode")) -> (x = y?=w88:bool)
    n45 = Compound Arithmetic op=OR(invert w89, w88) -> (w90:bool)
    n46 = case shown="True" w90 {
      tunnel: w96 -> [_ w98]
      tunnel: w93 -> [_ w97]
      frame False {
      }
      frame True {
        n47 = call <vilib>:"Bind Controls to SmartDashboard.vi"("Bound Control Refs"=w98, "Server IP Address"=w97) -> ()  [unwired: 10 in]
      }
    }
  }
  n48 = while {
    stop <- FALSE stop-if-true
    # "Default\nto normal vision"
    n49 = local read "Goal Camera Image"() -> (w101:T22)
    n50 = control-ref of="Goal Camera Image"() -> (w102:refnum<vi>)
    n51 = control-ref of="HSV Filter"() -> (w100:refnum<vi>)
    n52 = call "GoalVisionCalibrationHelper.vi"("HSV Filter"=w100, "Src Image"=w101, "Image Ctl Refnum"=w102) -> ()  [unwired: 9 in]
    n53 = Wait (ms)(milliseconds to wait=u32 100) -> ()  [unwired: 1 out]
  }
  n54 = while {
    tunnel: w40 -> [w112]
    tunnel: w39 -> [_]
    tunnel: [w113] -> _
    i -> [w113]
    stop <- FALSE stop-if-true
    # "Optionally read the DB image,\nlog, or retrieve images from a\nlogged match"
    n55 = local read "Camera IP"() -> (w105:string)
    n56 = local read "Rec Mode"() -> (w104:enum32{"Stop", "Record", "Playback"})
    n57 = call "624WPI_CameraRead MJPEG.vi"("Camera Settings"="Camera Settings", "Rec Mode"=w104, "Camera IP"=w105, "Enable"="Cam 1 Enable", "Refnum in"=w112) -> ("Active"=w109:bool, "Refnum out"=w111:T22, "FPS"=w108:dbl, "Bandwidth (Mbps)"=w107:dbl)  [unwired: 3 in]
    n58 = case shown="True" w109 {
      tunnel: w111 -> [_ w129]
      tunnel: w107 -> [_ w128]
      tunnel: w108 -> [_ w124]
      frame False {
        # "Sleep for 500ms"
        n59 = Wait Until Next ms Multiple(millisecond multiple=u32 500) -> ()  [unwired: 1 out]
      }
      frame True {
        w119 = TRUE ("Left Cam?")
        # "Use copy of image\nfor Goal Track"
        # "Update Mbps LED"
        n60 = case shown="4, 5" w128 {
          tunnel: [u32 6618880 ("Color Box") u32 16776722 ("Color Box") u32 16716800 ("Color Box")] -> w130
          frame Default {
          }
          frame 4, 5 {
          }
          frame 6.. {
          }
        }
        n61 = call "IMAQ Clear Overlay"("Image"=w129) -> ("error out"=w133:errorcluster, "Image Out"=w123:T22)  [unwired: 2 in, 7 out]
        n62 = Unbundle By Name(w133) -> ("status"=w134:bool)
        n63 = Bundle("Color Box"=w130, "Color Box"=w130) -> (w132:cluster{"Color Box":u32, "Color Box":u32})  [unwired: 1 out]
        n64 = property on="Image Message" class="Str"("Visible"=w134) -> ()  [unwired: 2 in, 2 out]
        n65 = Build Array(w132) -> (w131:cluster{"Color Box":u32, "Color Box":u32}[])
        n66 = local read "Score Cutoff"() -> (w125:dbl)
        n67 = property on="Mbps 2" class="Bool (strict)"("Colors [4]"=w131) -> ()  [unwired: 2 in, 2 out]
        n68 = local read "HSV Filter"() -> (w121:T25)
        n69 = local read "Vision Mode"() -> (w120:T19)
        n70 = call "Target Detection.vi"("Left Cam?"=w119, "Vision Mode"=w120, "Score Cutoff"=w125, "HSV Filter"=w121, "Src Image"=w123) -> ("Vision Targets"=w126:T34, "Annotated Image"=w117:T22, "Mask"=w116:T22)  [unwired: 3 in]
        n71 = call "Send Vision Packet.vi"("Camera"=i16 1, "Vision Targets"=w126) -> ()  [unwired: 14 in]
        n72 = call "Draw Vision Mode Overlay 624 Aerial Assist.vi"("Left Cam?"=w119, "Vision Mode"=w120, "Refnum in"=w117) -> ("Refnum out"=w118:T22)  [unwired: 8 in]
        "Camera Image" <- w118
        n73 = local read "Cam 1/2"() -> (w122:bool)
        n74 = case shown="False" w122 {
          tunnel: w118 -> [w136 _]
          tunnel: w116 -> [w135 _]
          frame False {
            # "Cam 1"
            "Goal Mask" <- w135
            "Goal Camera Image" <- w136
          }
          frame True {
            # "Cam 2"
          }
        }
        "Cam1 Mbps" <- w128
        "Cam1 FPS" <- w124
      }
    }
  }
  n75 = while {
    tunnel: w42 -> [w140]
    tunnel: w36 -> [w146]
    tunnel: w23 -> [w149]
    tunnel: [w147] -> _
    i -> [w147]
    stop <- FALSE stop-if-true
    # "These subVIs decode errors, user data, game mode, etc.\nOutputs aren't connected to indicators by default"
    n76 = call "624WPI_DashboardReceive DS Packet.vi"("Recv Socket"=w140) -> ("Battery"=w145:sgl, "Error Strings"=w144:string, "Robot IP Address"=w143:string, "Status"=w142:T35, "High Priority User Data"=w141:string)  [unwired: 5 in, 5 out]
    n77 = call <vilib>:"WPI_DashboardDecode Status Byte.vi"("Window Mode Notifier"=w149, "Status"=w142) -> ("Mode"=→"Mode":T30)  [unwired: 1 out]
    n78 = case shown="Default" w143 {
      selector: w143 -> [_ w152]
      tunnel: w146 -> [_ w153]
      tunnel: w144 -> [_ _]
      tunnel: w145 -> [_ _]
      tunnel: w141 -> [_ w151]
      frame "0.0.0.0" {
        # "DS not sending packets, or no robot exists yet.\nDon't poll the variables"
      }
      frame Default {
        # "Notify NT\nBind loop"
        # "DS sent a packet. use any data it\nprovided, poll others and update\ndisplays that don'teasily bind\nusing names"
        n79 = Send Notification(notification=w152, notifier=w153) -> ()  [unwired: 1 in, 2 out]
        "High Priority User Data" <- w151
      }
    }
  }
  n80 = while {
    tunnel: w19 -> [w164]
    tunnel: [w155] -> _
    i -> [w155]
    stop <- FALSE stop-if-true
    # "Optionally read the DB image,\nlog, or retrieve images from a\nlogged match"
    n81 = local read "Camera 2 IP"() -> (w158:string)
    n82 = local read "Rec Mode"() -> (w159:enum32{"Stop", "Record", "Playback"})
    n83 = local read "Camera Settings"() -> (w157:T21)
    n84 = call "624WPI_CameraRead MJPEG.vi"("Camera Settings"=w157, "Rec Mode"=w159, "Camera IP"=w158, "Enable"="Cam 2 Enable", "Refnum in"=w164) -> ("Active"=w163:bool, "Refnum out"=w162:T22, "FPS"=w161:dbl, "Bandwidth (Mbps)"=w160:dbl)  [unwired: 3 in]
    n85 = case shown="True" w163 {
      tunnel: w162 -> [_ w184]
      tunnel: w160 -> [_ w183]
      tunnel: w161 -> [_ w182]
      frame False {
        # "Sleep for 500ms"
        n86 = Wait Until Next ms Multiple(millisecond multiple=u32 500) -> ()  [unwired: 1 out]
      }
      frame True {
        w166 = FALSE ("Left Cam?")
        # "Update Mbps LED"
        n87 = call "IMAQ Clear Overlay"("Image"=w184) -> ("error out"=w181:errorcluster, "Image Out"=w172:T22)  [unwired: 2 in, 7 out]
        n88 = case shown="6.." w183 {
          tunnel: [u32 6618880 ("Color Box") u32 16776722 ("Color Box") u32 16716800 ("Color Box")] -> w179
          frame Default {
          }
          frame 4, 5 {
          }
          frame 6.. {
          }
        }
        n89 = Unbundle By Name(w181) -> ("status"=w180:bool)
        n90 = Bundle("Color Box"=w179, "Color Box"=w179) -> (w178:cluster{"Color Box":u32, "Color Box":u32})  [unwired: 1 out]
        n91 = property on="Image Message" class="Str"("Visible"=w180) -> ()  [unwired: 2 in, 2 out]
        n92 = Build Array(w178) -> (w177:cluster{"Color Box":u32, "Color Box":u32}[])
        n93 = property on="Cam2 LED" class="Bool (strict)"("Colors [4]"=w177) -> ()  [unwired: 2 in, 2 out]
        n94 = local read "HSV Filter"() -> (w170:T25)
        n95 = local read "Score Cutoff"() -> (w173:dbl)
        n96 = local read "Vision Mode"() -> (w167:T19)
        n97 = call "Target Detection.vi"("Left Cam?"=w166, "Vision Mode"=w167, "Score Cutoff"=w173, "HSV Filter"=w170, "Src Image"=w172) -> ("Vision Targets"=w174:T34, "Annotated Image"=w168:T22, "Mask"=w176:T22)  [unwired: 3 in]
        n98 = call "Send Vision Packet.vi"("Camera"=i16 2, "Vision Targets"=w174) -> ()  [unwired: 14 in]
        n99 = call "Draw Vision Mode Overlay 624 Aerial Assist.vi"("Left Cam?"=w166, "Vision Mode"=w167, "Refnum in"=w168) -> ("Refnum out"=w169:T22)  [unwired: 8 in]
        "Camera Image 2" <- w169
        n100 = local read "Cam 1/2"() -> (w171:bool)
        n101 = case shown="True" w171 {
          tunnel: w169 -> [_ w186]
          tunnel: w176 -> [_ w185]
          frame False {
            # "Cam 1"
          }
          frame True {
            # "Cam 2"
            n102 = local write "Goal Camera Image"(w186) -> ()
            n103 = local write "Goal Mask"(w185) -> ()
          }
        }
        "Cam2 Mbps" <- w183
        "Cam2 FPS" <- w182
      }
    }
  }
  n104 = control-ref of="Test Tree"() -> (w32:refnum<vi>)
  n105 = while {
    tunnel: w14 -> [w197]
    shift-right: [w196] -> _
    shift-left: w13 -> [w195]
    tunnel: [w194] -> _
    tunnel: w32 -> [w193]
    tunnel: w16 -> [w192]
    tunnel: w28 -> [w191]
    tunnel: w27 -> [_]
    tunnel: w21 -> [w190]
    i -> [w194]
    stop <- FALSE stop-if-true
    n106 = event shown="[0] Timeout" {
      selector: w191 -> [_ _ _ _ _ _ _ _ _ _ _ _ _ _ _ _]
      dyn-events: [_ _ _ _ _ _ _ _ _ _ _ _ _ w435 _ _] -> _
      timeout: u32 60 ("milliseconds to wait") -> [_ _ _ _ _ _ _ _ _ _ _ _ _ _ _ _]
      tunnel: w193 -> [w208 _ _ _ _ _ _ _ _ _ _ _ _ _ _ _]
      tunnel: "Test Tree" -> [_ _ _ _ _ _ _ _ w405 w412 w414 w418 w426 _ _ _]
      tunnel: w197 -> [_ w231 _ _ _ _ w368 w398 _ _ _ _ _ _ _ _]
      tunnel: [w202 w230 w329 w334 w342 w354 w367 w391 w404 w410 w413 w417 w425 w437 w451 w452] -> w196
      tunnel: w195 -> [w202 w230 w329 w334 w342 w354 w366 w391 w404 w410 w413 w417 w425 w437 w451 w452]
      tunnel: w192 -> [_ _ _ _ _ _ _ _ _ _ _ _ _ w438 _ w455]
      tunnel: w190 -> [_ _ _ _ _ _ _ _ _ _ _ _ _ w433 _ _]
      event Timeout {
        w207 = enum16{"Update", "Clear"}[] [enum."Clear", enum."Clear", enum."Clear", enum."Clear", enum."Update", enum."Update", enum."Clear"] items=["Update", "Clear"]
        n107 = event-data() -> ()  [unwired: 1 in, 1 out]
        n108 = local read "Mode"() -> (w205:T30)
        n109 = Index Array(array=w207, index=w205) -> (element=w206:enum16{"Update", "Clear"})
        n110 = call <vilib>:"NT Read String.vi"("Name"="TestMode/TestName") -> ("String"=w210:string)  [unwired: 9 in, 1 out]
        n111 = case shown="Default" w210 {
          tunnel: "TestMode/TestProgress" ("Name") -> [w224 _]
          tunnel: "TestMode/TestProgressText" ("Name") -> [w223 _]
          frame Default {
            n112 = call <vilib>:"NT Read Number.vi"("Name"=w224) -> ("Numeric"=w225:dbl)  [unwired: 9 in, 1 out]
            n113 = call <vilib>:"NT Read String.vi"("Name"=w223) -> ("String"=w226:string)  [unwired: 9 in, 1 out]
            n114 = Bundle("Numeric"=w225, "String"=w226) -> (→"Progress":cluster{"Numeric":dbl, "String":string})  [unwired: 1 in]
          }
          frame "" {
            n115 = property on="Progress" class="Clust (strict)"("Visible"=FALSE) -> ()  [unwired: 2 in, 2 out]
            n116 = local write "Test Name"(u16 0) -> ()
          }
        }
        n117 = case shown="\"Test\"" "Dashboard Tab" {
          tunnel: w208 -> [_ w220 _]
          tunnel: "/TestMode/Automatic/" ("Name Pattern") -> [_ w219 _]
          tunnel: w206 -> [_ w218 _]
          tunnel: w205 -> [_ w216 _]
          tunnel: [_ _ w222] -> _
          frame "Operation", Default {
          }
          frame "Test" {
            w215 = -2 ("Active Item:Row Number")
            n118 = call <vilib>:"NT Read and Format Entries as Tree.vi"("Operation"=w218, "Name Pattern"=w219, "Tree Refnum"=w220) -> ()  [unwired: 7 in, 2 out]
            n119 = Index Array(array=u32[] [14013909, 14013909, 14013909, 14013909, 14013909, 16777215, 14013909], index=w216) -> (element=w214:u32)
            n120 = property on="Test Tree" class="Tree (strict)"("Active Item Row Number"=w215, "ActiveColNum"=w215, "CellBG"=w214, "Active Item Row Number"=-1 ("Active Item:Row Number"), "CellBG"=u32 5789784 ("Color Box")) -> ()  [unwired: 2 in, 2 out]
          }
          frame "Variables" {
            n121 = control-ref of="Tree"() -> (w221:refnum<vi>)
            n122 = call <vilib>:"NT Read and Format Entries as Tree.vi"("Tree Refnum"=w221) -> ("Formatted Strings"=w222:cluster{"Name":string, "Value":string}[])  [unwired: 9 in, 1 out]
          }
        }
      }
      event "Test Tree": Value Change {
        # "Show appropriate\ncontrols"
        n123 = event-data() -> ("CtlRef"=w234:refnum<vi>, "NewVal"=w232:string)  [unwired: 1 in]
        n124 = call <vilib>:"WPI_UtilitiesGetTreeIOName.vi"("NewVal"=w232, "TreeControl in"=w234) -> ("I/O Name"=w235:string)  [unwired: 9 in]
        n125 = case shown="\"Camera\"" w235 {
          selector: w235 -> [_ w242 _ w260 w269 _]
          tunnel: w232 -> [_ _ w257 w259 _ w276]
          tunnel: w231 -> [_ _ _ _ _ w275]
          frame Default {
            w237 = FALSE ("Visible")
            w236 = FALSE ("Visible")
            n126 = property on="Motor" class="Clust (strict)"("Visible"=w236) -> ()  [unwired: 2 in, 2 out]
            n127 = property on="Test Ring" class="Ring (strict)"("Visible"=w236) -> ()  [unwired: 2 in, 2 out]
            n128 = property on="Rev/Fwd" class="Clust (strict)"("Visible"=w237) -> ()  [unwired: 2 in, 2 out]
            n129 = property on="On/Off" class="Bool (strict)"("Visible"=w237) -> ()  [unwired: 2 in, 2 out]
            n130 = property on="Test Slider" class="Slide (strict)"("Visible"=w237) -> ()  [unwired: 2 in, 2 out]
          }
          frame "Motor", "PWM" {
            w243 = FALSE ("Visible")
            n131 = case shown="\"Motor\", Default" w242 {
              tunnel: [1.0 ("Value") -1.0 ("Value")] -> w241
              tunnel: [255.0 ("Value") 1.0 ("Value")] -> w240
              tunnel: [128.0 ("Value") 0.0 ("Value")] -> w239
              tunnel: [64.0 ("Value") 0.5 ("Value")] -> w238
              frame "PWM" {
              }
              frame "Motor", Default {
              }
            }
            n132 = property on="Motor" class="Clust (strict)"("Visible"=TRUE) -> ()  [unwired: 2 in, 2 out]
            n133 = property on="Value" class="Slide (strict)"("Value"=w239, "Scale.Minimum"=w241, "Scale.Maximum"=w240, "Scale.Increment"=w238) -> ()  [unwired: 2 in, 2 out]
            n134 = property on="On/Off" class="Bool (strict)"("Visible"=w243) -> ()  [unwired: 2 in, 2 out]
            n135 = property on="Test Slider" class="Slide (strict)"("Visible"=w243) -> ()  [unwired: 2 in, 2 out]
            n136 = property on="Test Ring" class="Ring (strict)"("Visible"=w243) -> ()  [unwired: 2 in, 2 out]
            n137 = property on="Rev/Fwd" class="Clust (strict)"("Visible"=w243) -> ()  [unwired: 2 in, 2 out]
          }
          frame "Servo" {
            w255 = FALSE ("Visible")
            n138 = call <vilib>:"NT Read Number.vi"("Name"=w257) -> ("Numeric"=w256:dbl)  [unwired: 9 in, 1 out]
            n139 = property on="Test Slider" class="Slide (strict)"("Visible"=TRUE, "Scale.Maximum"=170.0 ("Scale.Range:Maximum")) -> ()  [unwired: 2 in, 2 out]
            n140 = local write "Test Slider"(w256) -> ()
            n141 = property on="Motor" class="Clust (strict)"("Visible"=w255) -> ()  [unwired: 2 in, 2 out]
            n142 = property on="Rev/Fwd" class="Clust (strict)"("Visible"=w255) -> ()  [unwired: 2 in, 2 out]
            n143 = property on="On/Off" class="Bool (strict)"("Visible"=w255) -> ()  [unwired: 2 in, 2 out]
            n144 = property on="Test Ring" class="Ring (strict)"("Visible"=w255) -> ()  [unwired: 2 in, 2 out]
          }
          frame "Relay", "Solenoid" {
            w258 = FALSE ("Visible")
            n145 = property on="Motor" class="Clust (strict)"("Visible"=w258) -> ()  [unwired: 2 in, 2 out]
            n146 = property on="Test Slider" class="Slide (strict)"("Visible"=w258) -> ()  [unwired: 2 in, 2 out]
            n147 = Search and Replace String(input string=w259, search string="/Value  **", replace string="/Direction") -> (result string=w265:string)  [unwired: 5 in, 3 out]
            n148 = property on="Test Ring" class="Ring (strict)"("Visible"=w258) -> ()  [unwired: 2 in, 2 out]
            n149 = call <vilib>:"NT Read String.vi"("Name"=w265) -> ("String"=w263:string)  [unwired: 9 in, 1 out]
            n150 = Equal?(x="Both directions", y=w263) -> (x = y?=w261:bool)
            n151 = Not(x=w261) -> (.not. x?=w262:bool)
            n152 = property on="Rev/Fwd" class="Clust (strict)"("Visible"=w261) -> ()  [unwired: 2 in, 2 out]
            n153 = property on="On/Off" class="Bool (strict)"("Visible"=w262, "Caption.Text"=w260) -> ()  [unwired: 2 in, 2 out]
          }
          frame "Compressor", "Digital Out" {
            w268 = FALSE ("Visible")
            # "Get direction and finish"
            n154 = property on="Motor" class="Clust (strict)"("Visible"=w268) -> ()  [unwired: 2 in, 2 out]
            n155 = property on="Test Slider" class="Slide (strict)"("Visible"=w268) -> ()  [unwired: 2 in, 2 out]
            n156 = property on="Test Ring" class="Ring (strict)"("Visible"=w268) -> ()  [unwired: 2 in, 2 out]
            n157 = property on="On/Off" class="Bool (strict)"("Visible"=TRUE, "Caption.Text"=w269) -> ()  [unwired: 2 in, 2 out]
            n158 = property on="Rev/Fwd" class="Clust (strict)"("Visible"=FALSE) -> ()  [unwired: 2 in, 2 out]
          }
          frame "Camera" {
            n159 = call <vilib>:"Get Last Path Segment.vi"("String in"=w276) -> ("String out"=w277:string)  [unwired: 10 in]
            n160 = property on="On/Off" class="Bool (strict)"("Visible"=FALSE) -> ()  [unwired: 2 in, 2 out]
            n161 = property on="Motor" class="Clust (strict)"("Visible"=FALSE) -> ()  [unwired: 2 in, 2 out]
            n162 = property on="Rev/Fwd" class="Clust (strict)"("Visible"=FALSE) -> ()  [unwired: 2 in, 2 out]
            n163 = case shown="\"Color Enable  **\"" w277 {
              tunnel: w276 -> [w283 w292 w301 w310 w319 _ w325]
              tunnel: w275 -> [w281 w289 w298 w307 w316 _ _]
              frame "Size  **" {
                n164 = Index Array(array=w281) -> (element=w280:cluster{string[]})  [unwired: 1 in]
                n165 = call <vilib>:"NT Read String.vi"("Name"=w283) -> ("String"=w282:string)  [unwired: 9 in, 1 out]
                n166 = Unbundle(w280) -> (w278:string[])
                n167 = Match First String(2:w278, 3:w282) -> (0:w279:i32)  [unwired: 1 out]
                n168 = property on="Test Ring" class="Ring (strict)"("Value"=w279, "Strings []"=w278) -> ()  [unwired: 2 in, 2 out]
                n169 = property on="Test Ring" class="Ring (strict)"("Visible"=TRUE) -> ()  [unwired: 2 in, 2 out]
                n170 = property on="Test Slider" class="Slide (strict)"("Visible"=FALSE) -> ()  [unwired: 2 in, 2 out]
              }
              frame "White Balance  **" {
                n171 = Index Array(array=w289, index=1) -> (element=w290:cluster{string[]})
                n172 = call <vilib>:"NT Read String.vi"("Name"=w292) -> ("String"=w291:string)  [unwired: 9 in, 1 out]
                n173 = Unbundle(w290) -> (w287:string[])
                n174 = Match First String(2:w287, 3:w291) -> (0:w286:i32)  [unwired: 1 out]
                n175 = property on="Test Ring" class="Ring (strict)"("Value"=w286, "Strings []"=w287) -> ()  [unwired: 2 in, 2 out]
                n176 = property on="Test Ring" class="Ring (strict)"("Visible"=TRUE) -> ()  [unwired: 2 in, 2 out]
                n177 = property on="Test Slider" class="Slide (strict)"("Visible"=FALSE) -> ()  [unwired: 2 in, 2 out]
              }
              frame "Exposure  **" {
                n178 = Index Array(array=w298, index=2) -> (element=w299:cluster{string[]})
                n179 = call <vilib>:"NT Read String.vi"("Name"=w301) -> ("String"=w300:string)  [unwired: 9 in, 1 out]
                n180 = Unbundle(w299) -> (w295:string[])
                n181 = Match First String(2:w295, 3:w300) -> (0:w296:i32)  [unwired: 1 out]
                n182 = property on="Test Ring" class="Ring (strict)"("Value"=w296, "Strings []"=w295) -> ()  [unwired: 2 in, 2 out]
                n183 = property on="Test Ring" class="Ring (strict)"("Visible"=TRUE) -> ()  [unwired: 2 in, 2 out]
                n184 = property on="Test Slider" class="Slide (strict)"("Visible"=FALSE) -> ()  [unwired: 2 in, 2 out]
              }
              frame "Exposure Priority  **" {
                n185 = Index Array(array=w307, index=3) -> (element=w308:cluster{string[]})
                n186 = call <vilib>:"NT Read String.vi"("Name"=w310) -> ("String"=w309:string)  [unwired: 9 in, 1 out]
                n187 = Unbundle(w308) -> (w304:string[])
                n188 = Match First String(2:w304, 3:w309) -> (0:w305:i32)  [unwired: 1 out]
                n189 = property on="Test Ring" class="Ring (strict)"("Value"=w305, "Strings []"=w304) -> ()  [unwired: 2 in, 2 out]
                n190 = property on="Test Ring" class="Ring (strict)"("Visible"=TRUE) -> ()  [unwired: 2 in, 2 out]
                n191 = property on="Test Slider" class="Slide (strict)"("Visible"=FALSE) -> ()  [unwired: 2 in, 2 out]
              }
              frame "Color Enable  **" {
                n192 = Index Array(array=w316, index=4) -> (element=w317:cluster{string[]})
                n193 = call <vilib>:"NT Read String.vi"("Name"=w319) -> ("String"=w318:string)  [unwired: 9 in, 1 out]
                n194 = Unbundle(w317) -> (w313:string[])
                n195 = Match First String(2:w313, 3:w318) -> (0:w314:i32)  [unwired: 1 out]
                n196 = property on="Test Ring" class="Ring (strict)"("Value"=w314, "Strings []"=w313) -> ()  [unwired: 2 in, 2 out]
                n197 = property on="Test Ring" class="Ring (strict)"("Visible"=TRUE) -> ()  [unwired: 2 in, 2 out]
                n198 = property on="Test Slider" class="Slide (strict)"("Visible"=FALSE) -> ()  [unwired: 2 in, 2 out]
              }
              frame Default {
                n199 = property on="Test Ring" class="Ring (strict)"("Visible"=FALSE) -> ()  [unwired: 2 in, 2 out]
                n200 = property on="Test Slider" class="Slide (strict)"("Visible"=FALSE) -> ()  [unwired: 2 in, 2 out]
              }
              frame "Brightness  **", "Color Level  **", "Compression  **", "FPS  **", "Sharpness  **" {
                n201 = call <vilib>:"NT Read Number.vi"("Name"=w325) -> ("Numeric"=w324:dbl)  [unwired: 9 in, 1 out]
                n202 = local write "Test Slider"(w324) -> ()
                n203 = property on="Test Slider" class="Slide (strict)"("Visible"=TRUE, "Scale.Maximum"=100.0 ("Scale.Range:Maximum")) -> ()  [unwired: 2 in, 2 out]
                n204 = property on="Test Ring" class="Ring (strict)"("Visible"=FALSE) -> ()  [unwired: 2 in, 2 out]
              }
            }
          }
        }
        n205 = property on="Progress" class="Clust (strict)"("Visible"=FALSE) -> ()  [unwired: 2 in, 2 out]
      }
      event "Test Name": Mouse Enter {
        # "Populate the ring with the list of tests"
        n206 = event-data() -> ()  [unwired: 1 in, 1 out]
        n207 = call <vilib>:"NT Read String Array.vi"("Name"="TestMode/TestList") -> ("String Array"=w333:string[])  [unwired: 9 in, 1 out]
        n208 = Build Array (concatenate)("Select the test to run...", w333) -> (w332:string[])
        n209 = property on="Test Name" class="Ring (strict)"("Strings []"=w332) -> ()  [unwired: 2 in, 2 out]
      }
      event "Test Name": Value Change {
        w335 = FALSE ("Visible")
        # "Tell the robot the test name to run"
        n210 = event-data() -> ("NewVal"=w339:u16)  [unwired: 1 in]
        n211 = property on="Test Name" class="Ring (strict)"() -> ("Strings []"=w340:string[])  [unwired: 2 in, 2 out]
        n212 = local write "Progress"(T23 {"Test Progress"=0, "Test Progress Text"=""} ("Progress")) -> ()
        n213 = Index Array(array=w340, index=w339) -> (element=w338:string)
        n214 = call <vilib>:"NT Write String.vi"("String"=w338, "Name"="TestMode/TestName") -> ()  [unwired: 9 in, 1 out]
        n215 = property on="Progress" class="Clust (strict)"("Visible"=TRUE) -> ()  [unwired: 2 in, 2 out]
        n216 = property on="Motor" class="Clust (strict)"("Visible"=w335) -> ()  [unwired: 2 in, 2 out]
        n217 = property on="Test Slider" class="Slide (strict)"("Visible"=w335) -> ()  [unwired: 2 in, 2 out]
        n218 = property on="On/Off" class="Bool (strict)"("Visible"=w335) -> ()  [unwired: 2 in, 2 out]
        n219 = property on="Rev/Fwd" class="Clust (strict)"("Visible"=w335) -> ()  [unwired: 2 in, 2 out]
        n220 = property on="Test Ring" class="Ring (strict)"("Visible"=w335) -> ()  [unwired: 2 in, 2 out]
      }
      event "Listbox": Double Click {
        n221 = event-data() -> ("PlatMods.Shift"=w343:bool, "Row"=w345:i32)  [unwired: 1 in]
        n222 = case shown="True" w343 {
          tunnel: w345 -> [w349 _]
          tunnel: 1 -> [w348 _]
          frame False {
            n223 = property on="Listbox" class="LstBox (strict)"() -> ("Item Symbols"=w347:i32[])  [unwired: 2 in, 2 out]
            n224 = Replace Array Subset(array=w347, new element=w348, index=w349) -> (w346:i32[])
            n225 = property on="Listbox" class="LstBox (strict)"("Item Symbols"=w346) -> ()  [unwired: 2 in, 2 out]
          }
          frame True {
            w350 = 0 ("Top Row")
            n226 = property on="Listbox" class="LstBox (strict)"() -> ("Number of Rows"=w352:u32)  [unwired: 2 in, 2 out]
            n227 = Initialize Array(0, w352) -> (w351:i32[])
            n228 = property on="Listbox" class="LstBox (strict)"("Top Row"=w350, "Value"=w350, "Item Symbols"=w351) -> ()  [unwired: 2 in, 2 out]
          }
        }
      }
      event "Listbox": Key Down {
        n229 = event-data() -> ("VKey"=w356:T36)  [unwired: 1 in]
        n230 = case shown="\"Left\", \"Right\"" w356 {
          selector: w356 -> [w361 _]
          tunnel: eventvkey."Left" ("VKey") -> [w359 _]
          frame "Left", "Right" {
            n231 = Equal?(x=w359, y=w361) -> (x = y?=w360:bool)
            n232 = Select(t=0, s=w360, f=1) -> (s? t:f=w362:i32)
            n233 = property on="Listbox" class="LstBox (strict)"() -> ("Item Symbols"=w365:i32[])  [unwired: 2 in, 2 out]
            n234 = Replace Array Subset(array=w365, new element=w362, index="Listbox") -> (w364:i32[])
            n235 = property on="Listbox" class="LstBox (strict)"("Item Symbols"=w364) -> ()  [unwired: 2 in, 2 out]
          }
          frame Default {
          }
        }
      }
      event "DB Camera Config": Value Change {
        n236 = event-data() -> ("NewVal"=w369:bool)  [unwired: 1 in]
        n237 = case shown="True" w369 {
          tunnel: w368 -> [w378 _]
          tunnel: [w371 w389] -> w367
          tunnel: w366 -> [w370 w389]
          frame False {
            w385 = "Camera"
            w388 = FALSE ("Visible")
            n238 = local read "Camera Settings"() -> (w377:T21)
            n239 = Index Array(array=w378) -> (element=w381:cluster{string[]})  [unwired: 1 in]
            n240 = Unbundle(w377) -> ("Frame Rate"=w376:i32, "Compression"=w375:i32, "Size"=w379:u16)
            n241 = Unbundle(w381) -> (w380:string[])
            n242 = Index Array(array=w380, index=w379) -> (element=w374:string)
            n243 = call-poly <vilib>:"Write Key.vi"("section"=w385, "value"=w374, "key"="Size", "refnum"=w370) -> ("refnum out"=w387:T32)  [unwired: 2 in, 5 out]
            n244 = call-poly <vilib>:"Write Key.vi"("section"=w385, "value"=w376, "key"="FrameRate", "refnum"=w387) -> ("refnum out"=w386:T32)  [unwired: 1 in, 6 out]
            n245 = property on="Camera Settings" class="Clust (strict)"("Visible"=w388) -> ()  [unwired: 2 in, 2 out]
            n246 = local write "DB Camera Config"(w388) -> ()
            n247 = call-poly <vilib>:"Write Key.vi"("section"=w385, "value"=w375, "key"="Compression", "refnum"=w386) -> ("refnum out"=w372:T32)  [unwired: 1 in, 6 out]
            n248 = call <vilib>:"Close Config Data.vi"("refnum"=w372) -> ("file path"=w373:path)  [unwired: 2 in, 8 out]
            n249 = call <vilib>:"Open Config Data.vi"("configuration file path"=w373) -> ("refnum"=w371:T32)  [unwired: 8 in, 2 out]
          }
          frame True {
            n250 = property on="Camera Settings" class="Clust (strict)"("Visible"=TRUE) -> ()  [unwired: 2 in, 2 out]
          }
        }
      }
      event "Camera Settings": Value Change {
        n251 = event-data() -> ("NewVal"=w402:T21)  [unwired: 1 in]
        n252 = Index Array(array=w398) -> (element=w397:cluster{string[]})  [unwired: 1 in]
        n253 = Unbundle(w402) -> ("Frame Rate"=w393:i32, "Compression"=w392:i32, "Size"=w395:u16)
        n254 = Unbundle(w397) -> (w396:string[])
        n255 = Index Array(array=w396, index=w395) -> (element=w394:string)
        n256 = Format Into String(format string="%s   %dfps   %d%%", w394, w393, w392) -> (resulting string=w399:string)  [unwired: 2 in, 1 out]
        n257 = Build Array(w399) -> (w400:string[])
        n258 = property on="DB Camera Config" class="Bool (strict)"("Strings [4]"=w400) -> ()  [unwired: 2 in, 2 out]
      }
      event "Motor": Value Change {
        n259 = event-data() -> ("NewVal.Enable"=w403:bool)  [unwired: 1 in]
        n260 = Unbundle("Motor") -> ("Value"=w408:dbl)  [unwired: 1 out]
        n261 = Select(t=w408, s=w403, f=0.0) -> (s? t:f=w406:dbl)
        n262 = call <vilib>:"NT Write Number.vi"("Numeric"=w406, "Name"=w405) -> ()  [unwired: 9 in, 1 out]
      }
      event "Test Slider": Value Change {
        n263 = event-data() -> ("NewVal"=w411:dbl)  [unwired: 1 in]
        n264 = call <vilib>:"NT Write Number.vi"("Numeric"=w411, "Name"=w412) -> ()  [unwired: 9 in, 1 out]
      }
      event "On/Off": Value Change {
        n265 = event-data() -> ("NewVal"=w416:bool)  [unwired: 1 in]
        n266 = Boolean To (0,1)(Boolean=w416) -> (0, 1=w415:i16)
        n267 = call <vilib>:"NT Write Number.vi"("Numeric"=w415, "Name"=w414) -> ()  [unwired: 9 in, 1 out]
      }
      event "Rev/Fwd": Value Change {
        n268 = event-data() -> ("NewVal.Forward"=w424:bool, "NewVal.Reverse"=w423:bool)  [unwired: 1 in]
        n269 = Boolean To (0,1)(Boolean=w424) -> (0, 1=w420:i16)
        n270 = Boolean To (0,1)(Boolean=w423) -> (0, 1=w422:i16)
        n271 = Negate(x=w422) -> (-x=w421:i16)
        n272 = Add(x=w420, y=w421) -> (x+y=w419:i16)
        n273 = call <vilib>:"NT Write Number.vi"("Numeric"=w419, "Name"=w418) -> ()  [unwired: 9 in, 1 out]
      }
      event "Test Ring": Value Change {
        n274 = event-data() -> ("NewVal"=w428:u16)  [unwired: 1 in]
        n275 = property on="Test Ring" class="Ring (strict)"() -> ("Strings []"=w429:string[])  [unwired: 2 in, 2 out]
        n276 = Index Array(array=w429, index=w428) -> (element=w427:string)
        n277 = call <vilib>:"NT Write String.vi"("String"=w427, "Name"=w426) -> ()  [unwired: 9 in, 1 out]
      }
      event "Rec Mode": Value Change {
        # "Update globals for recording mode and path to read log from.\nClear when logging and let NetworkTables set path for vision to\nuse."
        n278 = event-data() -> ("NewVal"=w439:enum32{"Stop", "Record", "Playback"})  [unwired: 1 in]
        n279 = case shown="\"Stop\", \"Record\"" w439 {
          tunnel: w438 -> [_ w441 w445]
          tunnel: [_ _ w449] -> w435
          tunnel: [_ _ w448] -> _
          tunnel: w433 -> [_ _ w443]
          tunnel: cluster{i32, i32} {-250, 170} -> [_ _ w442]
          tunnel: [_ _ T37 {"Image Size"=TRUE, "Image Type"=TRUE, "Pixel Value"=TRUE, "ROI Information"=TRUE, "Zoom Factor"=FALSE} ("Image Information Shown:All Elements")] -> w431
          tunnel: [_ _ TRUE ("Zoom Factor")] -> w430
          frame Default {
          }
          frame "Stop", "Record" {
            # "Place Window too"
            n280 = invoke class="VI" method="FP.Close"(reference=w441) -> (reference out=w440:refnum<vi>)  [unwired: 2 in, 2 out]
            n281 = invoke class="VI" method="Abort VI"(reference=w440) -> ()  [unwired: 2 in, 3 out]
          }
          frame "Playback" {
            n282 = call "Open Playback Panel.vi"("Offset"=w442, "DB VI Ref"=w443, "Playback in"=w445) -> ("Playback out"=w444:refnum<vi>)  [unwired: 8 in]
            n283 = register-events(w444) -> (reference out=w449:refnum<event-registration>, error out=w448:errorcluster)  [unwired: 2 in]
          }
        }
        n284 = global write "WPI_DashboardLogging Global.vi" "Recording"(w439) -> ()
        n285 = global write "WPI_DashboardLogging Global.vi" "Logging Filename"(path "") -> ()
        n286 = property on="Camera Image" class="ImageControl"("Image Information Shown"=w431, "Image Information Visible"=w430) -> ()  [unwired: 2 in, 2 out]
        n287 = call <vilib>:"WPI_DashboardNT Log FieldName Cache.vi"("Operation"=enum16{"Lookup/Add", "Index", "Clear"}."Clear") -> ()  [unwired: 8 in, 3 out]
      }
      event Panel Close {
        w450 = enum32{"Stop", "Record", "Playback"}."Stop" ("Rec Mode")
        n288 = event-data() -> ()  [unwired: 1 in, 4 out]
        n289 = local write "Rec Mode"(w450) -> ()
        n290 = global write "WPI_DashboardLogging Global.vi" "Recording"(w450) -> ()
      }
      event Panel Close {
        # "Abort playback window and ourself"
        n291 = event-data() -> ()  [unwired: 1 in, 4 out]
        n292 = invoke class="VI" method="FP.Close"(reference=w455) -> (reference out=w454:refnum<vi>)  [unwired: 2 in, 2 out]
        n293 = invoke class="VI" method="Abort VI"(reference=w454) -> (error out=w453:errorcluster)  [unwired: 2 in, 2 out]
        n294 = invoke class="VI" method="Abort VI"(error in=w453) -> ()  [unwired: 2 in, 3 out]
      }
    }
  }
  n295 = while {
    stop <- FALSE stop-if-true
    n296 = local read "Heartbeat"() -> (w465:dbl)
    n297 = local read "Pressure/Line"() -> (w457:dbl)
    n298 = Wait (ms)(milliseconds to wait=u32 1000) -> ()  [unwired: 1 out]
    n299 = call-poly "Change Detect.vi"("In"=w465) -> ("Changed?"=w458:bool)
    "Connection LED" <- w458
    n300 = Select(t=u32 6618880, s=w458, f=u32 16711680) -> (s? t:f=w466:u32)
    n301 = Less Or Equal?(x=w457, y=60.0) -> (x <= y?=w459:bool)
    n302 = Bundle(w466, w466) -> (w467:cluster{u32, u32})  [unwired: 1 in]
    n303 = Stop(stop? (T)="stop") -> ()
    n304 = property on="Pressure/Line" class="Slide (strict)"("Blinking"=w459) -> ()  [unwired: 2 in, 2 out]
    n305 = Build Array(w467, w467, w467, w467) -> (w468:cluster{u32, u32}[])
    n306 = property on="Connection LED" class="Bool (strict)"("Colors [4]"=w468) -> ()  [unwired: 2 in, 2 out]
  }
  n307 = while {
    stop <- FALSE stop-if-true
    # "Ghetto vision select radio buttons"
    n308 = event shown="[2] \"Extreme Right\": Mouse Up" {
      selector: _ -> [_ _ _]
      dyn-events: _ -> [_ _ _]
      timeout: _ -> [_ _ _]
      tunnel: [TRUE ("Normal Vision") _ _] -> w472
      tunnel: [_ TRUE ("Normal Vision") _] -> w471
      tunnel: [_ _ TRUE ("Normal Vision")] -> w470
      event "Normal Vision": Mouse Up {
        n309 = event-data() -> ()  [unwired: 1 in, 5 out]
      }
      event "Extreme Left": Mouse Up {
        n310 = event-data() -> ()  [unwired: 1 in, 5 out]
      }
      event "Extreme Right": Mouse Up {
        n311 = event-data() -> ()  [unwired: 1 in, 5 out]
      }
    }
    n312 = local write "Normal Vision"(w472) -> ()
    n313 = local write "Extreme Left"(w471) -> ()
    n314 = local write "Extreme Right"(w470) -> ()
  }
  n315 = property on="Test Ring" class="Ring (strict)"("Visible"=w33) -> ()  [unwired: 2 in, 2 out]
  n316 = property on="Motor" class="Clust (strict)"("Visible"=w33) -> ()  [unwired: 2 in, 2 out]
  n317 = property on="Progress" class="Clust (strict)"("Visible"=w33) -> ()  [unwired: 2 in, 2 out]
  n318 = property on="On/Off" class="Bool (strict)"("Visible"=w33) -> ()  [unwired: 2 in, 2 out]
  n319 = property on="Rev/Fwd" class="Clust (strict)"("Visible"=w33) -> ()  [unwired: 2 in, 2 out]
  n320 = property on="Camera Settings" class="Clust (strict)"("Visible"=w33) -> ()  [unwired: 2 in, 2 out]
  n321 = local write "DB Camera Config"(w33) -> ()
  n322 = disable-structure shown="Disabled" {
    frame Disabled {
      n323 = while {
        stop <- FALSE stop-if-true
        n324 = call "Field Drawing.vi"() -> ()  [unwired: 11 in, 1 out]
        n325 = Wait (ms)(milliseconds to wait=u32 100) -> ()  [unwired: 1 out]
      }
    }
    frame Enabled {
    }
  }
  n326 = global write "WPI_DashboardLogging Global.vi" "Recording"(w22) -> ()
  n327 = local write "Rec Mode"(w22) -> ()
  n328 = local write "Finish"(w10) -> ()
  n329 = local write "Abort"(w10) -> ()
  n330 = local write "Normal Vision"(TRUE ("Finish")) -> ()
  n331 = local write "Extreme Right"(w3) -> ()
  n332 = local write "Extreme Left"(w3) -> ()
  n333 = property on="Shooter" class="Clust (strict)"("Color"=w1) -> ()  [unwired: 2 in, 2 out]
  n334 = property on="Fieldcentric" class="Clust (strict)"("Color"=w1) -> ()  [unwired: 2 in, 2 out]
  n335 = property on="Roll" class="Clust (strict)"("Color"=w1) -> ()  [unwired: 2 in, 2 out]
  n336 = while {
    stop <- FALSE stop-if-true
    n337 = Select(t=Vision_Mode."Extreme Right" ("Vision Mode"), s="Extreme Right", f=Vision_Mode."Normal" ("Vision Mode")) -> (s? t:f=w489:T19)
    n338 = Select(t=Vision_Mode."Extreme Left" ("Vision Mode"), s="Extreme Left", f=w489) -> (s? t:f=w484:T19)
    n339 = Wait (ms)(milliseconds to wait=u32 200) -> ()  [unwired: 1 out]
    n340 = Bundle By Name(cluster=T39 {"Camera"={"Camera/View Angle X"=0.0, "Camera/Goal Track Timeout"=0.0, "Camera/View Angle Y"=0.0, "Camera/Goal Exposure"=0.0, "Camera/Vision Receive Timeout"=0.0, "Camera/Offset 1"=0.0, "Camera/Offset 2"=0.0}, "Gyro"={"Gyro/Angle Tolerance"=0.0, "Gyro/Steer Closeness Threshold"=0.0, "Steer PID"={"max"=0.0, "min"=0.0, "P"=0.0, "I"=0.0, "D"=0.0}, "Steer Close PID"={"max"=0.0, "min"=0.0, "P"=0.0, "I"=0.0, "D"=0.0}}, "Encoder"={"Encoders/Reset"=FALSE, "Encoders/Omni Constant"=0.0, "Encoders/Omni Tick Constant"=0.0, "Encoders/Left Constant"=0.0, "Encoders/Right Constant"=0.0, "Encoders/Right Tick Constant"=0.0}, "Auto Shift"={"AutoShift/Upshift Throttle Accel"=0.0, "AutoShift/Speed Threshold"=0.0, "AutoShift/Upshift Throttle"=0.0, "AutoShift/Upshift Accel"=0.0, "AutoShift/Downshift Accel"=0.0, "AutoShift/Downshift Throttle"=0.0, "AutoShift/Delay"=0.0, "AutoShift/Enabled"=FALSE}, "Auton"={"Auton/Left Shoot X-Coord"=0.0, "Auton/Right Shoot X-Coord"=0.0, "DistDrive/Distance Stop Threshold"=0.0, "DistDrive/Max Stop Speed"=0.0, "Auton/Back Piston Time"=0.0, "Auton/Manual Hot"=FALSE, "Auton/Manual Hot Right"=FALSE, "Default X PID"={"max"=0.0, "min"=0.0, "P"=0.0, "I"=0.0, "D"=0.0}, "Default Y PID"={"max"=0.0, "min"=0.0, "P"=0.0, "I"=0.0, "D"=0.0}, "Half Over Delay"=0.0}, "Drive/Ramp X"=0.0, "Drive/Ramp Y"=0.0, "Drive/Battery Cutoff"=0.0, "Pressure/Compressor Min Voltage"=0.0, "Pressure/Compressor Delay"=0.0, "Controller/Strafe Correction"=FALSE, "Shooter"={"Shooter/Reset Time"=0.0, "Shooter/Release Delay"=0.0, "Shooter/Pressure Steady Time"=0.0, "Shooter/Misfire Delay"=0.0, "Shooter/Ball Settle Time"=0.0, "Shooter/Line IR Delay"=0.0, "Pressure/Upper PSI Time"=0.0, "Pressure/Lower PSI Time"=0.0, "Shooter/Punch Delay"=0.0, "Shooter/Target Pressure"=0.0, "Pressure/Line B"=0.0, "Pressure/Line M"=0.0, "Pressure/Shooter M"=0.0, "Pressure/Shooter B"=0.0, "Halo Time"=0.0, "Soft Release Delay"=0.0, "Soft Unpin Delay"=0.0, "Soft Shoot Delay"=0.0, "Toss Release Time"=0.0}, "Rollers"={"Roller/Load IRs Verify Time"=0.0, "Roller/Center IR Latch Time"=0.0, "Roller/Speed Front"=0.0, "Roller/Speed Back"=0.0, "Roller/Entry Timeout"=0.0, "Roller/To Center Timeout"=0.0, "Roller/Sustain Time"=0.0, "Roller/Verify Center Time"=0.0}, "Abort"=FALSE, "Finish"=FALSE, "IR Halo Sustain Time"=0.0, "Disable Compressor"=FALSE, "Center Omni Drive Delay"=0, "Vision Mode"=enum."Normal", "Radius Throttle"=FALSE, "Fieldcentric"={"Relative Angle"=FALSE, "Point Robot"=FALSE, "X/Y ratio low"=0.0, "Steering Gain"=0.0, "Force Omni Down"=FALSE, "Enable"=FALSE, "X/Y ratio high"=0.0}, "Roll"={"X 1"=0.0, "Y 1"=0.0, "Y 2"=0.0, "X 2"=0.0, "Y 3"=0.0, "X 3"=0.0, "Time 1"=0, "Time 2"=0, "Time 3"=0, "Angle Start"=0.0, "Angle End"=0.0, "Angle Linearity"=0.0}, "Stick Deadband"=0.0} ("UDP Packet"), "Disable Compressor"="Disable Compressor", "Encoder"="Encoder", "Camera"="Camera", "Shooter"="Shooter", "Auton"="Auton", "Gyro"="Gyro", "Rollers"="Rollers", "Auto Shift"="Auto Shift", "Controller/Strafe Correction"="Controller/Strafe Correction", "Pressure/Compressor Min Voltage"="Pressure/Compressor Min Voltage", "Pressure/Compressor Delay"="Pressure/Compressor Delay", "Drive/Battery Cutoff"="Drive/Battery Cutoff", "Drive/Ramp Y"="Drive/Ramp Y", "Drive/Ramp X"="Drive/Ramp X", "Finish"="Finish", "Abort"="Abort", "IR Halo Sustain Time"="IR Halo Sustain Time", "Center Omni Drive Delay"="Center Omni Drive Delay", "Vision Mode"=w484, "Radius Throttle"="Radius Throttle", "Fieldcentric"="Fieldcentric", "Roll"="Roll", "Stick Deadband"="Stick Deadband") -> (w496:T39)
    n341 = Flatten To String(anything=w496) -> (data string=w479:string)  [unwired: 3 in, 2 out]
    n342 = Bundle By Name(cluster=T38 {"Type"=0, "data string"=""} ("output cluster"), "Type"=0, "data string"=w479) -> (w493:T38)
    n343 = String Length(string=w479) -> ()  [unwired: 1 out]
    n344 = call "Send Omni Packet.vi"("output cluster"=w493) -> ()  [unwired: 11 in]
  }
  n345 = local write "Prefs Status"("") -> ()
  n346 = local write "Reload"(TRUE ("Reload")) -> ()
  n347 = property on="Prefs Status" class="Str"("Visible"=FALSE, "Blinking"=FALSE) -> ()  [unwired: 2 in, 2 out]
  n348 = while {
    shift-right: [w523] -> _
    shift-left: _ -> [w522]
    stop <- FALSE stop-if-true
    w552 = cluster{u32, u32} {5898228, 5898228}
    # "Log gyro data for maneuver graph"
    # "c"
    # "c"
    # "Drive"
    n349 = Wait (ms)(milliseconds to wait=u32 100) -> ()  [unwired: 1 out]
    n350 = disable-structure shown="Enabled" {
      disable-tunnel: [w658 w682] -> w519
      disable-tunnel: [w656 w677] -> w573
      disable-tunnel: [w652 w680] -> w572
      disable-tunnel: [w650 w676] -> w571
      disable-tunnel: [w648 w675] -> w524
      disable-tunnel: [w646 w673] -> w569
      disable-tunnel: [w645 w683] -> w568
      disable-tunnel: [w642 w672] -> w565
      disable-tunnel: [w641 w671] -> w564
      disable-tunnel: [w638 w684] -> w558
      disable-tunnel: [w637 w678] -> w557
      disable-tunnel: [w632 w679] -> w517
      disable-tunnel: [w630 w674] -> w556
      disable-tunnel: [w628 w681] -> w554
      disable-tunnel: [_ w669] -> w525
      disable-tunnel: [_ w668] -> w521
      frame Disabled {
        # "c"
        # "c"
        # "c"
        # "c"
        # "c"
        # "c"
        # "c"
        # "c"
        # "c"
        n351 = call <vilib>:"SD Read String.vi"("Name"="Drive Indicators") -> ("String"=w666:string)  [unwired: 8 in, 2 out]
        n352 = call <vilib>:"SD Read String.vi"("Name"="Auton Indicators") -> ("String"=w663:string)  [unwired: 8 in, 2 out]
        n353 = call <vilib>:"SD Read String.vi"("Name"="Roller Indicators") -> ("String"=w661:string)  [unwired: 8 in, 2 out]
        n354 = call <vilib>:"SD Read Number.vi"("Name"="Gyro/Steer Target") -> ("Numeric"=w650:dbl)  [unwired: 8 in, 2 out]
        n355 = call <vilib>:"SD Read String.vi"("Name"="Encoder Indicators") -> ("String"=w639:string)  [unwired: 8 in, 2 out]
        n356 = call <vilib>:"SD Read Boolean.vi"("Name"="IR Dist/Line Detected Right") -> ("Boolean"=w641:bool)  [unwired: 8 in, 2 out]
        n357 = call <vilib>:"SD Read Boolean.vi"("Name"="IR Dist/Line Detected Left") -> ("Boolean"=w642:bool)  [unwired: 8 in, 2 out]
        n358 = call <vilib>:"SD Read Number.vi"("Name"="Heartbeat") -> ("Numeric"=w630:dbl)  [unwired: 8 in, 2 out]
        n359 = call <vilib>:"SD Read Boolean.vi"("Name"="Gyro/In Range") -> ("Boolean"=w646:bool)  [unwired: 8 in, 2 out]
        n360 = call <vilib>:"SD Read Number.vi"("Name"="Gyro Heading") -> ("Numeric"=w648:dbl)  [unwired: 8 in, 2 out]
        n361 = call <vilib>:"SD Read String.vi"("Name"="Auton/Files") -> ("String"=w656:string)  [unwired: 8 in, 2 out]
        n362 = call <vilib>:"SD Read String.vi"("Name"="Halo/Indicators") -> ("String"=w634:string)  [unwired: 8 in, 2 out]
        n363 = call <vilib>:"SD Read Number.vi"("Name"="100ms Loop Time") -> ("Numeric"=w637:dbl)  [unwired: 8 in, 2 out]
        n364 = call <vilib>:"SD Read String.vi"("Name"="Shooter/Indicators") -> ("String"=w653:string)  [unwired: 8 in, 2 out]
        n365 = Unflatten From String(type=T8 {"Halo"=FALSE, "Roller Halo"=FALSE, "Shooter Halo"=FALSE, "Auto Halo"=FALSE, "Manual Halo"=FALSE} ("Halo Indicators"), binary string=w634) -> (value=w632:T8)  [unwired: 3 in, 2 out]
        n366 = Unflatten From String(type=T14 {"Avg Distance L/R"=0.0, "Avg Speed L/R"=0.0, "Left"={"Distance"=0.0, "Speed"=0.0, "Ticks"=0.0}, "Right"={"Distance"=0.0, "Speed"=0.0, "Ticks"=0.0}, "Omni"={"Distance"=0.0, "Speed"=0.0, "Ticks"=0.0}} ("Encoder Data"), binary string=w639) -> (value=w628:T14)  [unwired: 3 in, 2 out]
        n367 = Unflatten From String(type=T7 {"Drive/Throttle"=0.0, "Drive/Steer"=0.0, "Drive/Translation X"=0.0, "Drive/Omni"=FALSE, "Roller/Front Output"=0.0, "Roller/Back Output"=0.0, "Roller/Front Solenoid"=FALSE, "Roller/Back Solenoid"=FALSE, "Drive/Gear"=0.0} ("Drive Indicators"), binary string=w666) -> (value=w638:T7)  [unwired: 3 in, 2 out]
        n368 = Unflatten From String(type=T13 {"Pressure/Line"=-1.0, "Pressure/Shooter"=-1.0, "Shooter/Release"=FALSE, "Shooter/Trigger"=FALSE, "Shooter/Retracted"=FALSE, "Shooter/Ready"=FALSE, "Shooter/Add"=FALSE, "Shooter/State"=enum."Wait", "Shooter/Punch"=FALSE, "Shooter/High"=FALSE, "Shooter/AutoPunch"=FALSE} ("Shooter Indicators"), binary string=w653) -> (value=w652:T13)  [unwired: 3 in, 2 out]
        n369 = Unflatten From String(type=T18 {"DistDrive/Steer"=FALSE, "DistDrive/Y Check"=FALSE, "Auton/Left Hot"=FALSE, "Auton/Right Hot"=FALSE, "DistDrive/Y Dist"=0.0, "DistDrive/Y Target"=0.0, "DistDrive/X Dist"=0.0, "DistDrive/X Target"=0.0, "Gyro Heading"=0.0, "DistDrive/Steer Target"=0.0, "DistDrive/X Check"=FALSE, "Auton/Hot Found"=FALSE, "Auton/Goals Used"=0.0, "Auton/Total Commands"=0.0, "Auton/Current Command"=0.0, "Auton/File"=0.0} ("Auton Indicators"), binary string=w663) -> (value=w645:T18)  [unwired: 3 in, 2 out]
        n370 = Unflatten From String(type=T5 {"Roller/Front IR"=FALSE, "Roller/Center IR"=FALSE, "Roller/Back IR"=FALSE, "Roller/IR State"=enum."Waiting", "Roller/Auto Enabled"=FALSE, "Roller/Hold"=FALSE, "Roller/Net Solenoid"=FALSE} ("Roller Indicators"), binary string=w661) -> (value=w658:T5)  [unwired: 3 in, 2 out]
      }
      frame Enabled {
        n371 = local read "High Priority User Data"() -> (w687:string)
        n372 = Unflatten From String(type=T40 {"Gyro/Steer Target"=0.0, "Gyro/In Range"=FALSE, "Gyro Heading"=0.0, "Auton/Files"="", "Auton Indicators"={"DistDrive/Steer"=FALSE, "DistDrive/Y Check"=FALSE, "Auton/Left Hot"=FALSE, "Auton/Right Hot"=FALSE, "DistDrive/Y Dist"=0.0, "DistDrive/Y Target"=0.0, "DistDrive/X Dist"=0.0, "DistDrive/X Target"=0.0, "Gyro Heading"=0.0, "DistDrive/Steer Target"=0.0, "DistDrive/X Check"=FALSE, "Auton/Hot Found"=FALSE, "Auton/Goals Used"=0.0, "Auton/Total Commands"=0.0, "Auton/Current Command"=0.0, "Auton/File"=0.0}, "Heartbeat"=0.0, "100ms Loop Time"=0, "IR Dist/Line Detected Left"=FALSE, "IR Dist/Line Detected Right"=FALSE, "Roller Indicators"={"Roller/Front IR"=FALSE, "Roller/Center IR"=FALSE, "Roller/Back IR"=FALSE, "Roller/IR State"=enum."Waiting", "Roller/Auto Enabled"=FALSE, "Roller/Hold"=FALSE, "Roller/Net Solenoid"=FALSE}, "Shooter/Indicators"={"Pressure/Line"=0.0, "Pressure/Shooter"=0.0, "Shooter/Release"=FALSE, "Shooter/Trigger"=FALSE, "Shooter/Retracted"=FALSE, "Shooter/Ready"=FALSE, "Shooter/Add"=FALSE, "Shooter/State"=enum."Wait", "Shooter/Punch"=FALSE, "Shooter/High"=FALSE, "Shooter/AutoPunch"=FALSE}, "Halo/Indicators"={"Halo"=FALSE, "Roller Halo"=FALSE, "Shooter Halo"=FALSE, "Auto Halo"=FALSE, "Manual Halo"=FALSE}, "Drive Indicators"={"Drive/Throttle"=0.0, "Drive/Steer"=0.0, "Drive/Translation X"=0.0, "Drive/Omni"=FALSE, "Roller/Front Output"=0.0, "Roller/Back Output"=0.0, "Roller/Front Solenoid"=FALSE, "Roller/Back Solenoid"=FALSE, "Drive/Gear"=0.0}, "Encoder Data"={"Avg Distance L/R"=0.0, "Avg Speed L/R"=0.0, "Left"={"Distance"=0.0, "Speed"=0.0, "Ticks"=0.0}, "Right"={"Distance"=0.0, "Speed"=0.0, "Ticks"=0.0}, "Omni"={"Distance"=0.0, "Speed"=0.0, "Ticks"=0.0}}, "Vision Mode "=enum."Normal", "Drivetrain Mode"=enum."Manual"} ("Indicator Packet"), binary string=w687) -> (value=w685:T40, error out=w670:errorcluster)  [unwired: 3 in, 1 out]
        n373 = Unbundle By Name(w685) -> ("Drive Indicators"=w684:T7, "Auton Indicators"=w683:T18, "Roller Indicators"=w682:T5, "Encoder Data"=w681:T14, "Shooter/Indicators"=w680:T13, "Halo/Indicators"=w679:T8, "100ms Loop Time"=w678:i32, "Auton/Files"=w677:string, "Gyro/Steer Target"=w676:dbl, "Gyro Heading"=w675:dbl, "Heartbeat"=w674:dbl, "Gyro/In Range"=w673:bool, "IR Dist/Line Detected Left"=w672:bool, "IR Dist/Line Detected Right"=w671:bool, "Vision Mode"=w669:T19, "Drivetrain Mode"=w668:T29)
        n374 = call <vilib>:"Clear Errors.vi"("error in (no error)"=w670) -> ()  [unwired: 6 in, 1 out]
      }
    }
    "Gyro Heading" <- w524
    "Auton/Files" <- w573
    "Gyro/Steer Target" <- w571
    "Gyro/In Range" <- w569
    "IR Dist/Line Detected Right" <- w564
    "IR Dist/Line Detected Left" <- w565
    "Gyro Heading" <- w524
    "Shooter Indicators" <- w572
    "Auton Indicators" <- w568
    "Roller Indicators" <- w519
    "Roller Indicators 2" <- w519
    "Drive Indicators" <- w558
    "Drive Indicators 2" <- w558
    "Time/100ms loop exec time" <- w557
    "Halo Indicators" <- w517
    "Heartbeat" <- w556
    "Encoder Data" <- w554
    "Halo Indicators 2" <- w517
    "Gyro Heading" <- w524
    "Vision Mode" <- w525
    "Vision Mode Cam" <- w525
    "Vision Mode Goal Tab" <- w525
    "Drivetrain Mode" <- w521
    n375 = call-poly "Change Detect.vi"("In"=w521) -> ("Changed?"=w520:bool)
    n376 = case shown="\"Manual\", Default" w521 {
      tunnel: w524 -> [_ w578]
      tunnel: [w574 w577] -> w523
      tunnel: w522 -> [w574 w576]
      tunnel: w520 -> [_ w575]
      frame "Manual", Default {
        # "Leave array alone\nto display it"
      }
      frame "Roll Maneuver", "Alt Roll Maneuver" {
        n377 = case shown="True" w575 {
          tunnel: w578 -> [w581 w583]
          tunnel: [w580 w582] -> w577
          tunnel: w576 -> [w579 _]
          frame False {
            n378 = Build Array (concatenate)(w579, w581) -> (w580:dbl[])
          }
          frame True {
            # "start a new array"
            n379 = Build Array(w583) -> (w582:dbl[])
          }
        }
      }
    }
    "Maneuver Gyro Data" <- w523
    n380 = Unbundle By Name(w568) -> ("Auton/Left Hot"=→"Auton/Left Hot":bool, "Auton/Right Hot"=→"Auton/Right Hot":bool)
    n381 = Unbundle By Name(w572) -> ("Shooter/Retracted"=→"Shooter Retracted":bool, "Shooter/State"=w544:T1, "Shooter/Ready"=w543:bool, "Shooter/Add"=→"Shooter/Add":bool, "Shooter/Release"=→"Shooter/Release":bool, "Shooter/Trigger"=→"Shooter/Trigger":bool, "Shooter/High"=w541:bool, "Pressure/Line"=w549:dbl, "Pressure/Shooter"=→"Pressure/Shooter" →"Pressure/Shooter":dbl)  [unwired: 2 out]
    "Shooter/Ready" <- w543
    "Shooter/State" <- w544
    "Pressure/Line" <- w549
    "Shooter/High" <- w541
    n382 = Unbundle By Name(w517) -> ("Auto Halo"=→"Halo Mode":bool)
    n383 = Unbundle By Name(w519) -> ("Roller/Auto Enabled"=→"Roller Mode":bool)
    n384 = disable-structure shown="Enabled" {
      disable-tunnel: w549 -> [w693 _]
      disable-tunnel: [w691 "PSI Good"] -> w548
      disable-tunnel: w544 -> [w690 _]
      disable-tunnel: w543 -> [w689 _]
      disable-tunnel: [w690 "Shooter State"] -> w527
      disable-tunnel: [w689 "Shooter Ready"] -> w537
      disable-tunnel: w541 -> [w688 _]
      disable-tunnel: [w688 "Shooter High"] -> w526
      frame Enabled {
        n385 = Greater?(x=w693, y="Low PSI") -> (0:w691:bool)
      }
      frame Disabled {
      }
    }
    n386 = Unbundle By Name(w558) -> ("Drive/Gear"=→"Drive/Gear":dbl)
    n387 = Tick Count (ms)() -> (millisecond timer value=w531:u32)
    n388 = Quotient & Remainder(x=w531, y=u32 450) -> (x-y*floor(x/y)=w532:u32)  [unwired: 1 out]
    n389 = Less Or Equal?(x=w532, y=u32 250) -> (x <= y?=w533:bool)
    n390 = call "Signal Timer.vi"("Input"=w548, "Edge"=FALSE ("x < y?"), "Interval"=500.0, "Pull"=TRUE) -> ("Filtered Output"=w535:bool)  [unwired: 11 in]
    n391 = Not(x=w535) -> (.not. x?=w536:bool)
    n392 = And(x=w536, y=w533) -> (x .and. y?=w534:bool)
    n393 = case shown="False" w534 {
      tunnel: [w590 w627] -> w539
      tunnel: [w586 w626] -> w528
      tunnel: w527 -> [w587 _]
      tunnel: w537 -> [w588 _]
      tunnel: w526 -> [w584 _]
      tunnel: w535 -> [w585 _]
      tunnel: u32 16711680 -> [w589 w626]
      tunnel: "TANK LOW" -> [w591 w627]
      frame False {
        n394 = case shown="\"Toss Prep\"" w587 {
          tunnel: [w593 w607 "FIRE!!!" "Reload..." "TOSS" w623] -> w590
          tunnel: [w597 w603 u32 16318208 u32 11862255 u32 10854655 w625] -> w586
          tunnel: w585 -> [_ _ _ _ _ w622]
          tunnel: w588 -> [w592 w601 _ _ _ _]
          tunnel: w584 -> [_ w600 _ _ _ _]
          tunnel: w591 -> [_ _ _ _ _ w620]
          tunnel: w589 -> [_ _ _ _ _ w619]
          frame "Soft Release" {
            n395 = Select(t=u32 5898228, s=w592, f=u32 14869218) -> (s? t:f=w597:u32)
            n396 = Select(t="SOFT Ready", s=w592, f="SOFT  ______") -> (s? t:f=w593:string)
          }
          frame "Fill Piston" {
            n397 = Select(t=u32 16740882, s=w600, f=u32 6618880) -> (s? t:f=w599:u32)
            n398 = Select(t=w599, s=w601, f=u32 14869218) -> (s? t:f=w603:u32)
            n399 = Select(t="High", s=w600, f="Low") -> (s? t:f=w606:string)
            n400 = Select(t=" Ready", s=w601, f="  ______") -> (s? t:f=w608:string)
            n401 = Concatenate Strings(w606, w608) -> (w607:string)
          }
          frame "Lift Halo", "Trigger", "Soft Unpin".."Soft Shoot" {
          }
          frame "Reset" {
          }
          frame "Toss Prep" {
          }
          frame Default {
            n402 = Select(t=u32 9151100, s=w622, f=w619) -> (s? t:f=w625:u32)
            n403 = Select(t="Pressure OK", s=w622, f=w620) -> (s? t:f=w623:string)
          }
        }
      }
      frame True {
        # "Pressure Low overrides all others"
      }
    }
    n404 = Bundle(cluster=w552, w528, w528) -> (w551:cluster{u32, u32})
    n405 = Bundle(cluster=w552, w528, w528) -> (w550:cluster{u32, u32})
    n406 = Build Array(w551, w550) -> (w542:cluster{u32, u32}[])
    n407 = property on="Shooter State Indicator" class="Bool (strict)"("Colors [4]"=w542, "BoolText.Text"=w539) -> ()  [unwired: 2 in, 2 out]
    "Shooter State Indicator" <- FALSE ("Shooter State Indicator")
  }
  n408 = while {
    shift-right: [w698] -> _
    shift-left: w4 -> [w704]
    stop <- FALSE stop-if-true
    n409 = flat-sequence {
      tunnel: ["Save"] -> w710
      tunnel: ["Reload"] -> w708
      tunnel: [w714] -> w700
      tunnel: w710 -> [w719]
      tunnel: [w719] -> w709
      tunnel: w708 -> [w718]
      tunnel: [w718] -> w707
      tunnel: w700 -> [w717]
      tunnel: [w717] -> w699
      tunnel: w709 -> [w722]
      tunnel: w707 -> [w723]
      tunnel: [w721] -> w706
      tunnel: w699 -> [w720]
      frame #0 {
        n410 = control-ref of="Dashboard Tab"() -> (w714:refnum<vi>)
      }
      frame #1 {
      }
      frame #2 {
        n411 = Or(x=w722, y=w723) -> (x .or. y?=w721:bool)
        n412 = case shown="True" w721 {
          tunnel: w722 -> [w732 _]
          tunnel: w720 -> [w727 _]
          frame True {
            n413 = flat-sequence {
              tunnel: w727 -> [w736]
              tunnel: w732 -> [w737]
              tunnel: [w737] -> w726
              tunnel: [w736] -> w725
              tunnel: [w746] -> w731
              tunnel: [w752] -> w730
              tunnel: [w739] -> w729
              tunnel: [w747] -> w728
              tunnel: w726 -> [w756]
              tunnel: w725 -> [w743]
              tunnel: [w738] -> w724
              tunnel: w731 -> [w769]
              tunnel: w730 -> [w766]
              tunnel: w729 -> [w765]
              tunnel: w728 -> [w763]
              tunnel: w724 -> [w761]
              frame #0 {
                n414 = local write "Prefs Status"("") -> ()
                n415 = property on="Prefs Status" class="Str"("Visible"=FALSE) -> ()  [unwired: 2 in, 2 out]
                n416 = Wait (ms)(milliseconds to wait=u32 500) -> ()  [unwired: 1 out]
              }
              frame #1 {
                w755 = -1  # All Pages
                n417 = call <vilib>:"Get Tab Control Refs.vi"("Page Index"=w755, "TabControl in"=w743) -> ("ControlsOnPage"=w754:refnum<vi>[])  [unwired: 9 in]
                n418 = Select(t=enum16{"Save", "Load"}."Save" ("Operation"), s=w756, f=enum16{"Save", "Load"}."Load" ("Operation")) -> (s? t:f=w745:enum16{"Save", "Load"})
                n419 = call "Open Preferences File.vi"("Operation"=w745) -> ("File refnum out"=w746:T32)  [unwired: 8 in, 2 out]
                n420 = case shown="\"Save\"" w745 {
                  tunnel: ["loaded" ("string") "saved" ("string")] -> w749
                  frame "Load" {
                  }
                  frame "Save" {
                  }
                }
                n421 = call "624_Get All Control References.vi"("Controls[] in"=w754) -> ("Warnings List"=w740:string, "Named Controls"=w741:T41)  [unwired: 8 in, 1 out]
                n422 = call "Goal Vision Preferences.vi"("Named Controls in"=w741, "Operation"=w745, "Refnum"=w746) -> ("Count"=w744:i32, "Warnings List"=w742:string)  [unwired: 7 in]
                n423 = call "UDP Packet Preferences.vi"("Named Controls in"=w741, "Operation"=w745, "Refnum"=w746) -> ("Count"=w751:i32, "Warnings List"=w753:string)  [unwired: 7 in]
                n424 = Concatenate Strings(w742, w753, w740) -> (w752:string)
                n425 = Compound Arithmetic op=ADD(w744, w751) -> (w739:i32)
                n426 = Number To Decimal String(number=w739) -> (decimal integer string=w748:string)  [unwired: 1 in]
                n427 = Concatenate Strings(w748, " preferences " ("string"), w749) -> (w747:string)
                n428 = Greater Than 0?(x=w739) -> (x > 0?=w738:bool)
              }
              frame #2 {
                n429 = case shown="False" w761 {
                  tunnel: [u32 16711680 u32 6618880] -> w762
                  frame False {
                    n430 = One Button Dialog(message="Prefs file missing or empty. Copy from git to C:\\Users\\Public\\624_dashboard_prefs.txt") -> ()  [unwired: 1 in, 1 out]
                  }
                  frame True {
                  }
                }
                n431 = call <vilib>:"Close Config Data.vi"("refnum"=w769) -> ()  [unwired: 9 in, 2 out]
                n432 = local write "Reload"(FALSE ("Reload")) -> ()
                n433 = local write "Save"(FALSE ("Save")) -> ()
                n434 = property on="Prefs Status" class="Str"("Visible"=TRUE, "Text.BGColor"=w762) -> ()  [unwired: 2 in, 2 out]
                "Warnings List" <- w766
                "Preferences Count" <- w765
                "Prefs Status" <- w763
              }
            }
          }
          frame False {
            n435 = Wait (ms)(milliseconds to wait=u32 250) -> ()  [unwired: 1 out]
          }
        }
      }
    }
    n436 = Increment(x=w704) -> (x+1=w703:i32)
    n437 = Select(t=0 ("Counter"), s=w706, f=w703) -> (s? t:f=w698:i32)
    n438 = Greater Or Equal?(x=w698, y=20) -> (x >= y?=w701:bool)
    n439 = case shown="True" w701 {
      frame False {
      }
      frame True {
        # "Reset Status indicator"
        n440 = property on="Prefs Status" class="Str"("Visible"=FALSE) -> ()  [unwired: 2 in, 2 out]
        n441 = local write "Prefs Status"("") -> ()
      }
    }
  }
  n442 = while {
    stop <- FALSE stop-if-true
    w785 = 0.0 ("X Scale.Range:Minimum")
    w786 = 0
    w787 = 10 ("Timestep(ms)")
    # "Bundle up the planned angle path\nand a graph of the actual angle data \nto show simultaneously on the graph"
    n443 = local read "Roll"() -> (w781:T27)
    n444 = Wait (ms)(milliseconds to wait=u32 1000) -> ()  [unwired: 1 out]
    n445 = call "Build Roll Maneuver.vi"("Roll"=w781, "Timestep(ms)"=w787) -> ("Total Time"=w783:i32, "Angle Array"=w788:dbl[], "Y Array"=w794:dbl[], "X Array"=w795:dbl[])  [unwired: 6 in]
    n446 = Build Array(w795, w794) -> (w793:dbl[][])
    n447 = Build Array(w783) -> (w782:i32[])
    n448 = Add(x=w783, y=100) -> (x+y=w784:i32)
    n449 = Bundle(w786, "Timestep(ms)"=w787, w793) -> (→"Drive Graph":cluster{i32, "Timestep(ms)":i32, dbl[][]})  [unwired: 1 in]
    n450 = Bundle(w786, "Timestep(ms)"=w787, "Angle Array"=w788) -> (w775:T42)  [unwired: 1 in]
    n451 = property on="Drive Graph" class="WFGraph (strict)"("XScale.Maximum"=w784, "XScale.Minimum"=w785, "XScale.MarkerVals[]"=w782) -> ()  [unwired: 2 in, 2 out]
    n452 = property on="Angle Graph" class="WFGraph (strict)"("XScale.Maximum"=w784, "XScale.Minimum"=w785, "XScale.MarkerVals[]"=w782, "YScale.MarkerVals[]"=dbl[] [180.0, 135.0, 90.0, 45.0, 0.0, -45.0, -90.0, -135.0, -180.0] ("Y Scale.Marker Values[]")) -> ()  [unwired: 2 in, 2 out]
    n453 = local read "Maneuver Gyro Data"() -> (w779:dbl[])
    n454 = Bundle(0, 100, "Maneuver Gyro Data"=w779) -> (w776:cluster{i32, i32, "Maneuver Gyro Data":dbl[]})  [unwired: 1 in]
    n455 = Build Array(w775, w776) -> (→"Angle Graph":T26)
  }
